vi "Verification.vi"(1 "appended array 2":string[][](array[string])) -> (0 "Array":i32[][](array[numeric]))   [LabVIEW 2019]
panel:
  in  "Blank Button 48":bool
  in  "Blank Button 47":bool
  in  "Blank Button 46":bool
  in  "Blank Button 45":bool
  in  "Blank Button 44":bool
  in  "Blank Button 43":bool
  in  "Blank Button 42":bool
  in  "Blank Button 41":bool
  in  "Color Box 45":u32(colorbox)
  in  "Color Box 46":u32(colorbox)
  in  "Color Box 48":u32(colorbox)
  in  "Color Box 43":u32(colorbox)
  in  "Color Box 41":u32(colorbox)
  in  "Color Box 42":u32(colorbox)
  in  "Color Box 44":u32(colorbox)
  in  "Color Box 47":u32(colorbox)
  in  "Blank Button 40":bool
  in  "Blank Button 39":bool
  in  "Color Box 40":u32(colorbox)
  in  "Color Box 39":u32(colorbox)
  in  "Blank Button 38":bool
  in  "Blank Button 37":bool
  in  "Color Box 38":u32(colorbox)
  in  "Color Box 37":u32(colorbox)
  in  "Blank Button 36":bool
  in  "Blank Button 35":bool
  in  "Color Box 36":u32(colorbox)
  in  "Color Box 35":u32(colorbox)
  in  "Blank Button 34":bool
  in  "Blank Button 33":bool
  in  "Color Box 34":u32(colorbox)
  in  "Color Box 33":u32(colorbox)
  in  "Blank Button 32":bool
  in  "Blank Button 31":bool
  in  "Color Box 32":u32(colorbox)
  in  "Color Box 31":u32(colorbox)
  in  "Blank Button 30":bool
  in  "Blank Button 29":bool
  in  "Color Box 30":u32(colorbox)
  in  "Color Box 29":u32(colorbox)
  in  "Blank Button 28":bool
  in  "Blank Button 27":bool
  in  "Color Box 28":u32(colorbox)
  in  "Color Box 27":u32(colorbox)
  in  "Blank Button 26":bool
  in  "Blank Button 25":bool
  in  "Color Box 26":u32(colorbox)
  in  "Color Box 25":u32(colorbox)
  in  "Blank Button 24":bool
  in  "Blank Button 23":bool
  in  "Blank Button 22":bool
  in  "Blank Button 21":bool
  in  "Blank Button 20":bool
  in  "Blank Button 19":bool
  in  "Blank Button 18":bool
  in  "Blank Button 17":bool
  in  "Color Box 24":u32(colorbox)
  in  "Color Box 22":u32(colorbox)
  in  "Color Box 21":u32(colorbox)
  in  "Color Box 19":u32(colorbox)
  in  "Color Box 23":u32(colorbox)
  in  "Color Box 18":u32(colorbox)
  in  "Color Box 17":u32(colorbox)
  in  "Color Box 20":u32(colorbox)
  in  "Blank Button 16":bool
  in  "Blank Button 15":bool
  in  "Blank Button 14":bool
  in  "Blank Button 13":bool
  in  "Blank Button 12":bool
  in  "Blank Button 11":bool
  in  "Blank Button 10":bool
  in  "Blank Button 9":bool
  in  "Color Box 16":u32(colorbox)
  in  "Color Box 14":u32(colorbox)
  in  "Color Box 11":u32(colorbox)
  in  "Color Box 13":u32(colorbox)
  in  "Color Box 9":u32(colorbox)
  in  "Color Box 15":u32(colorbox)
  in  "Color Box 12":u32(colorbox)
  in  "Color Box 10":u32(colorbox)
  in  "Blank Button 8":bool
  in  "Blank Button 7":bool
  in  "Blank Button 6":bool
  in  "Blank Button 5":bool
  in  "Blank Button 2":bool
  in  "Blank Button":bool
  in  "Color Box 2":u32(colorbox)
  in  "Color Box":u32(colorbox)
  in  "Blank Button 4":bool
  in  "Blank Button 3":bool
  in  "Color Box 4":u32(colorbox)
  in  "Color Box 3":u32(colorbox)
  in  "Color Box 8":u32(colorbox)
  in  "Color Box 5":u32(colorbox)
  in  "Color Box 6":u32(colorbox)
  in  "Color Box 7":u32(colorbox)
  in  "stop":bool
  in  "Blanc":dbl
  in  "Vert":dbl
  in  "Bleu":dbl
  in  "Orange":dbl
  in  "Jaune":dbl
  in  "Rouge":dbl
  # "Vérification des couleurs"
  # "W"
  # "R"
  # "B"
  # "G"
  # "Y"
  # "O"
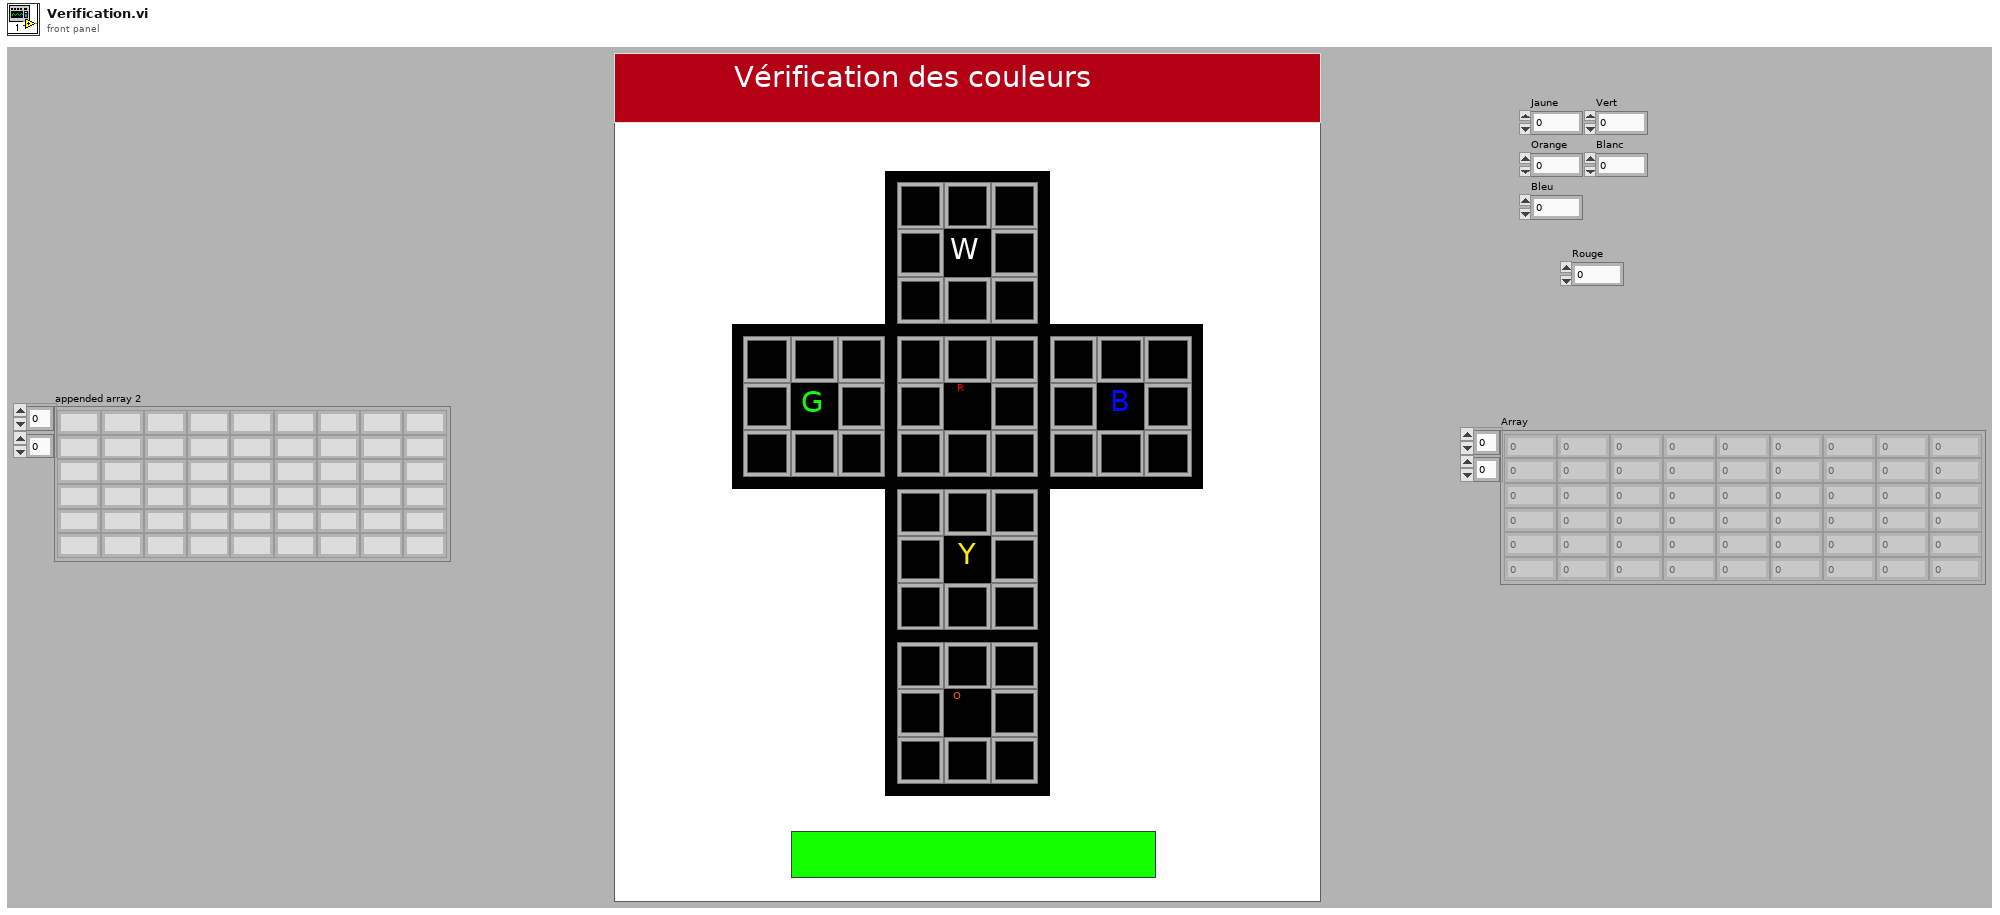
[diagram p1: front panel]
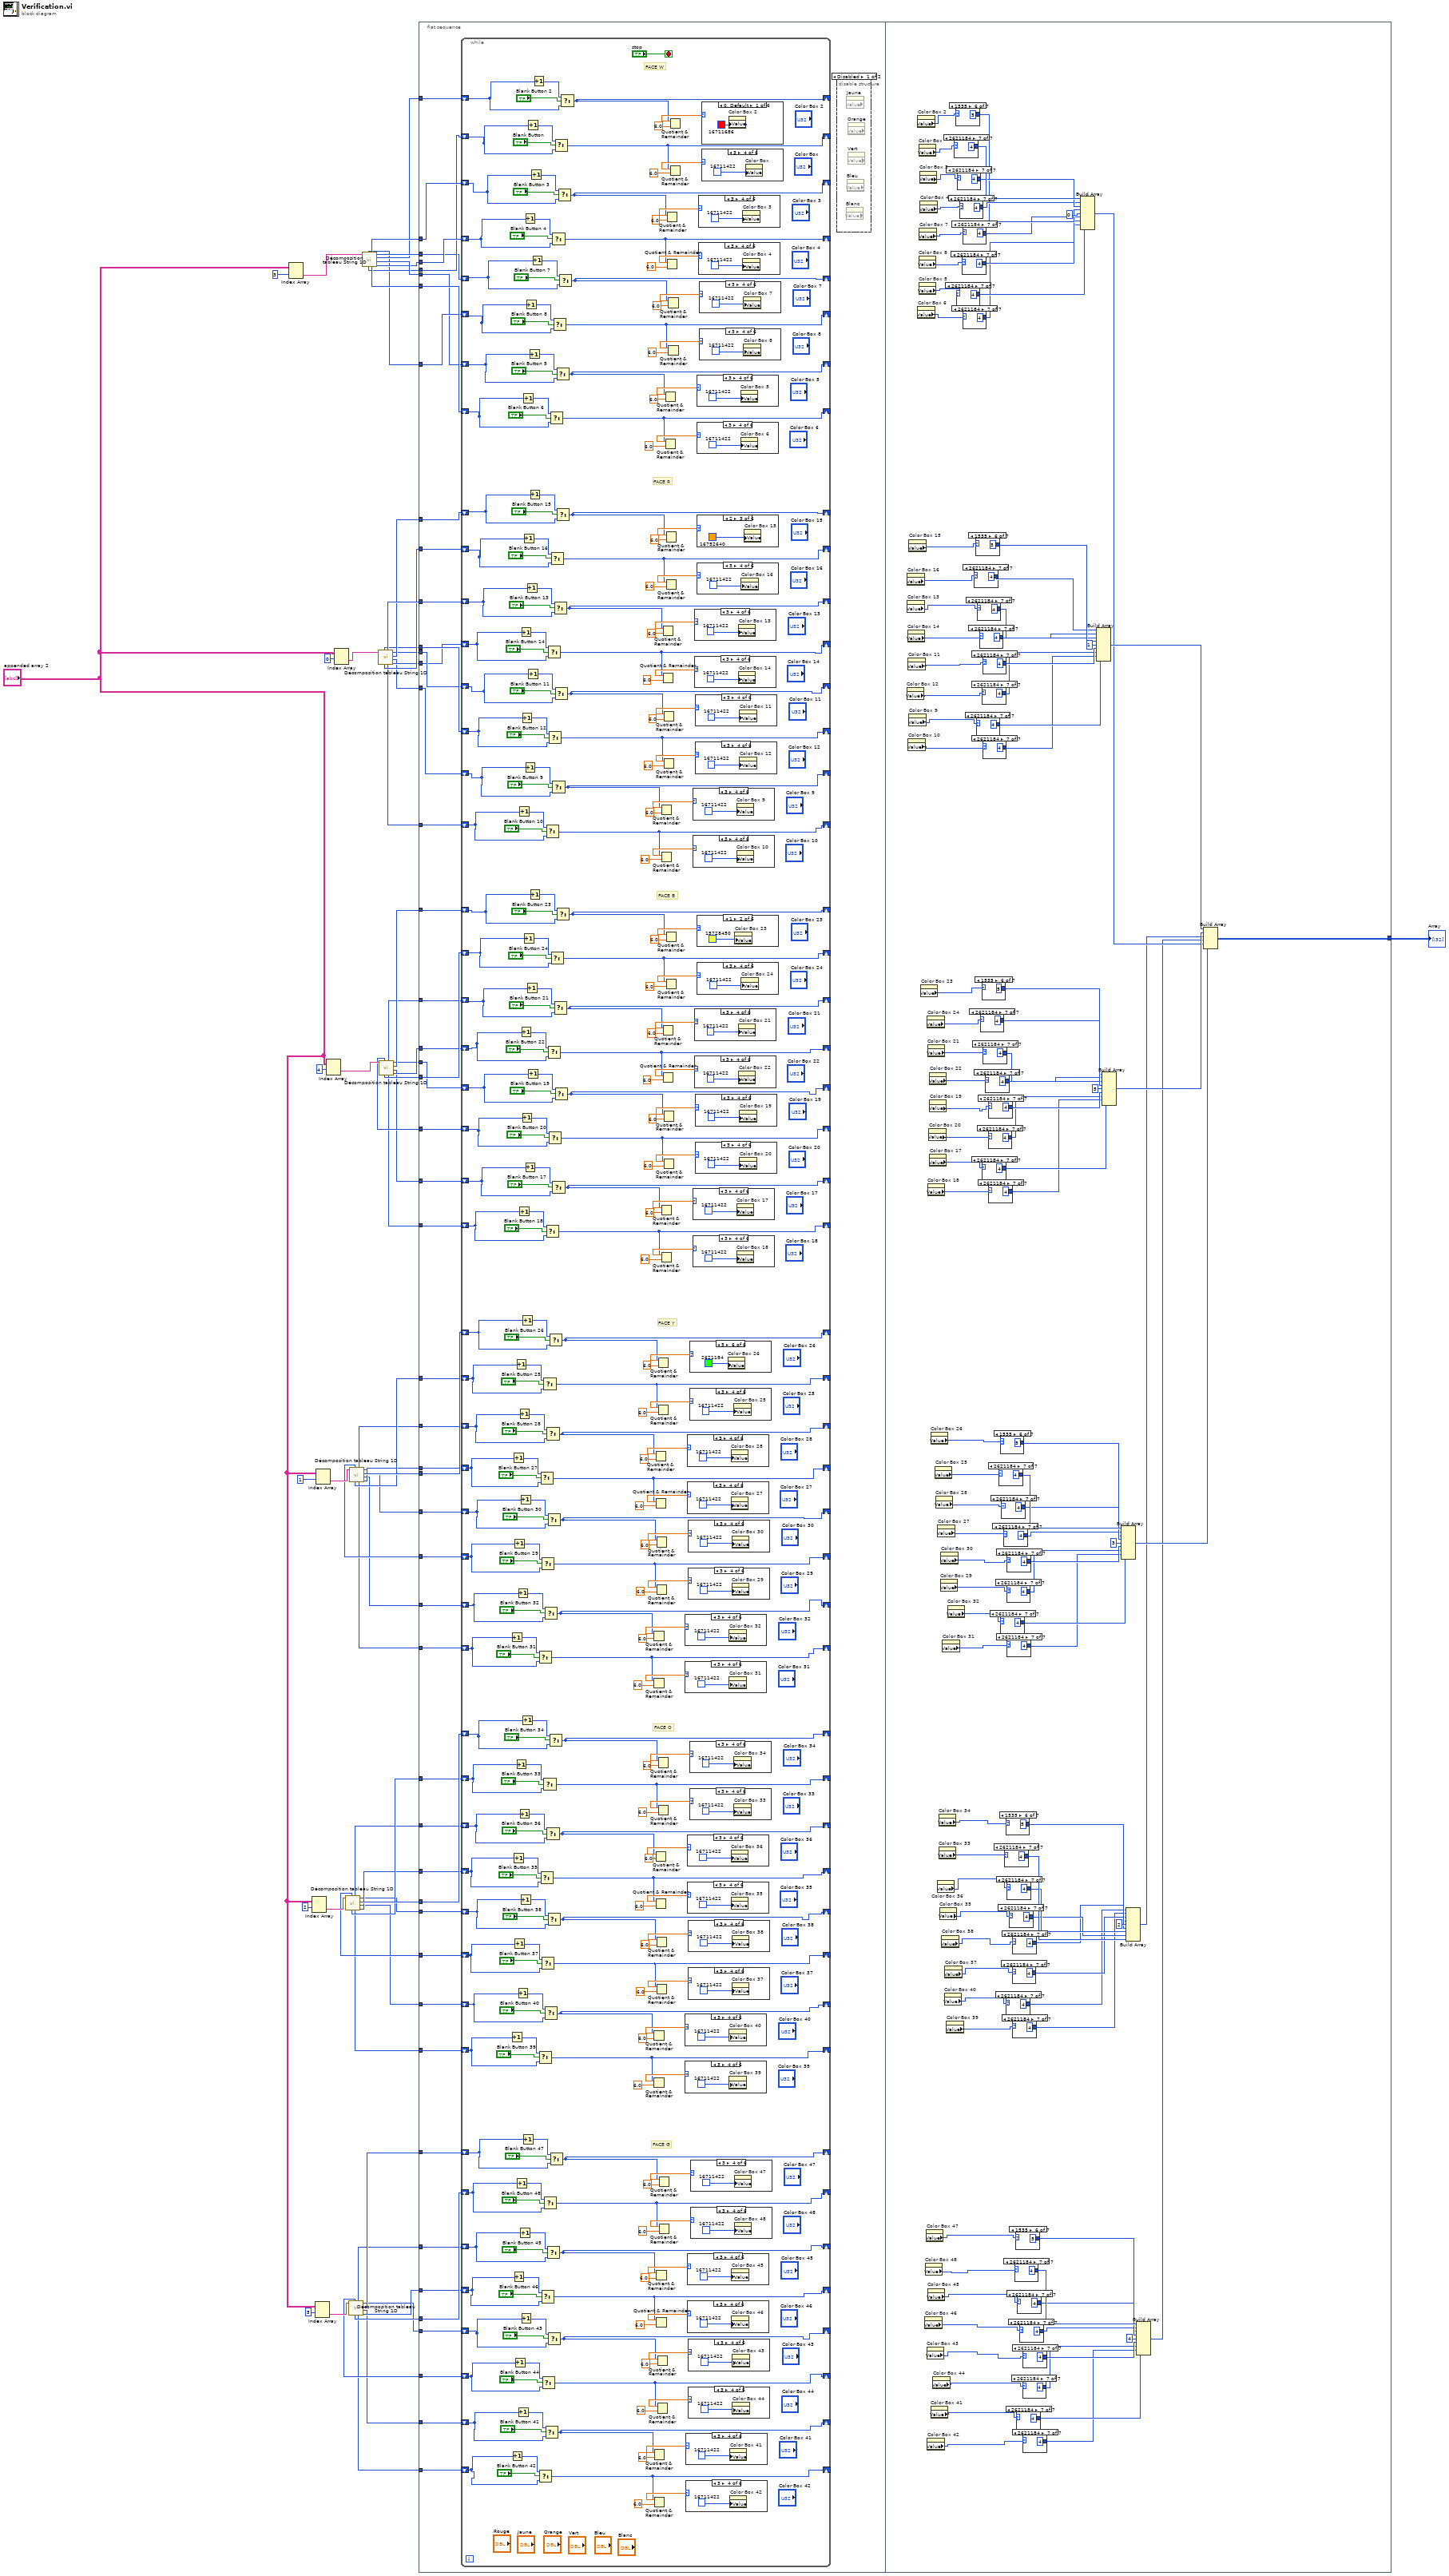
[diagram p0: block diagram]
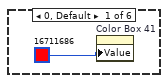
[diagram p3: hidden frame]
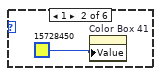
[diagram p4: hidden frame]
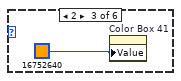
[diagram p5: hidden frame]
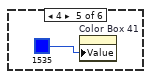
[diagram p6: hidden frame]
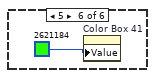
[diagram p7: hidden frame]
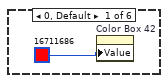
[diagram p8: hidden frame]
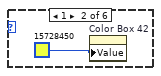
[diagram p9: hidden frame]
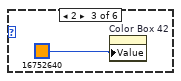
[diagram p10: hidden frame]
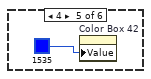
[diagram p11: hidden frame]
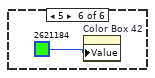
[diagram p12: hidden frame]
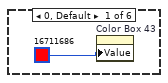
[diagram p13: hidden frame]
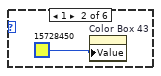
[diagram p14: hidden frame]
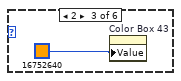
[diagram p15: hidden frame]
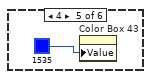
[diagram p16: hidden frame]
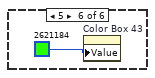
[diagram p17: hidden frame]
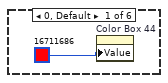
[diagram p18: hidden frame]
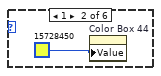
[diagram p19: hidden frame]
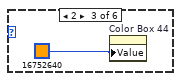
[diagram p20: hidden frame]
diagram:
  n1 = Index Array(array="appended array 2", index (row)=3) -> (element=w61:string[])  [unwired: 1 in]
  n2 = Index Array(array="appended array 2", index (row)=2) -> (element=w37:string[])  [unwired: 1 in]
  n3 = Index Array(array="appended array 2", index (row)=5) -> (element=w38:string[])  [unwired: 1 in]
  n4 = Index Array(array="appended array 2", index (row)=1) -> (element=w36:string[])  [unwired: 1 in]
  n5 = Index Array(array="appended array 2", index (row)=4) -> (element=w41:string[])  [unwired: 1 in]
  n6 = Index Array(array="appended array 2", index (row)=0) -> (element=w52:string[])  [unwired: 1 in]
  n7 = call "Décomposition tableau String 1D.vi"("appended array in"=w37) -> ("7"=w22:i32, "6"=w19:i32, "4"=w25:i32, "3"=w21:i32, "8"=w18:i32, "2"=w23:i32, "9"=w24:i32, "1"=w20:i32)  [unwired: 3 in]
  n8 = call "Décomposition tableau String 1D.vi"("appended array in"=w38) -> ("7"=w30:i32, "6"=w27:i32, "4"=w33:i32, "3"=w29:i32, "8"=w26:i32, "2"=w31:i32, "9"=w32:i32, "1"=w28:i32)  [unwired: 3 in]
  n9 = call "Décomposition tableau String 1D.vi"("appended array in"=w36) -> ("7"=w14:i32, "6"=w11:i32, "4"=w17:i32, "3"=w13:i32, "8"=w10:i32, "2"=w15:i32, "9"=w16:i32, "1"=w12:i32)  [unwired: 3 in]
  n10 = call "Décomposition tableau String 1D.vi"("appended array in"=w61) -> ("7"=w57:i32, "6"=w58:i32, "4"=w54:i32, "3"=w59:i32, "8"=w56:i32, "2"=w60:i32, "9"=w55:i32, "1"=w51:i32)  [unwired: 3 in]
  n11 = call "Décomposition tableau String 1D.vi"("appended array in"=w52) -> ("7"=w47:i32, "6"=w44:i32, "4"=w49:i32, "3"=w46:i32, "8"=w43:i32, "2"=w50:i32, "9"=w48:i32, "1"=w45:i32)  [unwired: 3 in]
  n12 = call "Décomposition tableau String 1D.vi"("appended array in"=w41) -> ("7"=w6:i32, "6"=w3:i32, "4"=w9:i32, "3"=w5:i32, "8"=w2:i32, "2"=w7:i32, "9"=w8:i32, "1"=w4:i32)  [unwired: 3 in]
  n13 = flat-sequence {
    tunnel: w60 -> [w110]
    tunnel: w59 -> [w105]
    tunnel: w57 -> [w109]
    tunnel: w56 -> [w108]
    tunnel: w55 -> [w107]
    tunnel: w54 -> [w106]
    tunnel: w51 -> [w104]
    tunnel: w58 -> [w103]
    tunnel: w43 -> [w102]
    tunnel: w45 -> [w101]
    tunnel: w49 -> [w100]
    tunnel: w48 -> [w99]
    tunnel: w46 -> [w98]
    tunnel: w47 -> [w97]
    tunnel: w50 -> [w96]
    tunnel: w44 -> [w95]
    tunnel: w33 -> [w94]
    tunnel: w32 -> [w93]
    tunnel: w31 -> [w92]
    tunnel: w30 -> [w91]
    tunnel: w29 -> [w90]
    tunnel: w28 -> [w89]
    tunnel: w27 -> [w88]
    tunnel: w26 -> [w87]
    tunnel: w25 -> [w86]
    tunnel: w24 -> [w85]
    tunnel: w23 -> [w84]
    tunnel: w22 -> [w83]
    tunnel: w21 -> [w82]
    tunnel: w20 -> [w81]
    tunnel: w19 -> [w80]
    tunnel: w18 -> [w79]
    tunnel: w17 -> [w78]
    tunnel: w16 -> [w77]
    tunnel: w15 -> [w76]
    tunnel: w14 -> [w75]
    tunnel: w13 -> [w74]
    tunnel: w12 -> [w73]
    tunnel: w11 -> [w72]
    tunnel: w10 -> [w71]
    tunnel: w9 -> [w70]
    tunnel: w8 -> [w69]
    tunnel: w7 -> [w68]
    tunnel: w6 -> [w67]
    tunnel: w5 -> [w66]
    tunnel: w4 -> [w65]
    tunnel: w3 -> [w64]
    tunnel: w2 -> [w63]
    tunnel: [w796] -> w1
    frame #0 {
      n14 = while {
        shift-right: [w392] -> _
        shift-left: w106 -> [w389]
        shift-right: [w390] -> _
        shift-left: w107 -> [w396]
        shift-right: [w377] -> _
        shift-left: w110 -> [w378]
        shift-right: [w375] -> _
        shift-left: w109 -> [w376]
        shift-right: [w356] -> _
        shift-left: w105 -> [w351]
        shift-right: [w355] -> _
        shift-left: w104 -> [w352]
        shift-right: [w354] -> _
        shift-left: w103 -> [w357]
        shift-right: [w353] -> _
        shift-left: w108 -> [w358]
        shift-right: [w317] -> _
        shift-left: w100 -> [w318]
        shift-right: [w316] -> _
        shift-left: w99 -> [w309]
        shift-right: [w315] -> _
        shift-left: w96 -> [w308]
        shift-right: [w314] -> _
        shift-left: w97 -> [w307]
        shift-right: [w313] -> _
        shift-left: w98 -> [w306]
        shift-right: [w312] -> _
        shift-left: w101 -> [w305]
        shift-right: [w311] -> _
        shift-left: w95 -> [w304]
        shift-right: [w310] -> _
        shift-left: w102 -> [w303]
        shift-right: [w270] -> _
        shift-left: w70 -> [w262]
        shift-right: [w269] -> _
        shift-left: w69 -> [w261]
        shift-right: [w268] -> _
        shift-left: w68 -> [w260]
        shift-right: [w267] -> _
        shift-left: w67 -> [w259]
        shift-right: [w266] -> _
        shift-left: w66 -> [w258]
        shift-right: [w265] -> _
        shift-left: w65 -> [w257]
        shift-right: [w264] -> _
        shift-left: w64 -> [w256]
        shift-right: [w263] -> _
        shift-left: w63 -> [w255]
        shift-right: [w168] -> _
        shift-left: w78 -> [w163]
        shift-right: [w167] -> _
        shift-left: w77 -> [w164]
        shift-right: [w166] -> _
        shift-left: w76 -> [w165]
        shift-right: [w169] -> _
        shift-left: w75 -> [w162]
        shift-right: [w170] -> _
        shift-left: w74 -> [w161]
        shift-right: [w171] -> _
        shift-left: w73 -> [w160]
        shift-right: [w172] -> _
        shift-left: w72 -> [w159]
        shift-right: [w173] -> _
        shift-left: w71 -> [w174]
        shift-right: [w189] -> _
        shift-left: w86 -> [w190]
        shift-right: [w188] -> _
        shift-left: w85 -> [w181]
        shift-right: [w187] -> _
        shift-left: w84 -> [w180]
        shift-right: [w186] -> _
        shift-left: w83 -> [w177]
        shift-right: [w185] -> _
        shift-left: w82 -> [w179]
        shift-right: [w184] -> _
        shift-left: w81 -> [w178]
        shift-right: [w183] -> _
        shift-left: w80 -> [w176]
        shift-right: [w182] -> _
        shift-left: w79 -> [w175]
        shift-right: [w126] -> _
        shift-left: w94 -> [w124]
        shift-right: [w123] -> _
        shift-left: w93 -> [w125]
        shift-right: [w122] -> _
        shift-left: w92 -> [w111]
        shift-right: [w121] -> _
        shift-left: w91 -> [w112]
        shift-right: [w120] -> _
        shift-left: w90 -> [w113]
        shift-right: [w119] -> _
        shift-left: w89 -> [w114]
        shift-right: [w118] -> _
        shift-left: w88 -> [w115]
        shift-right: [w117] -> _
        shift-left: w87 -> [w116]
        stop <- "stop" stop-if-true
        # "FACE G"
        # "FACE O"
        # "FACE Y"
        # "FACE B"
        # "FACE R"
        # "FACE W"
        n15 = Increment(x=w174) -> (x+1=w240:i32)
        n16 = Increment(x=w175) -> (x+1=w205:i32)
        n17 = Increment(x=w116) -> (x+1=w144:i32)
        n18 = Increment(x=w162) -> (x+1=w237:i32)
        n19 = Increment(x=w177) -> (x+1=w208:i32)
        n20 = Increment(x=w112) -> (x+1=w141:i32)
        n21 = Increment(x=w160) -> (x+1=w253:i32)
        n22 = Increment(x=w178) -> (x+1=w192:i32)
        n23 = Increment(x=w114) -> (x+1=w157:i32)
        n24 = Increment(x=w164) -> (x+1=w224:i32)
        n25 = Increment(x=w181) -> (x+1=w221:i32)
        n26 = Increment(x=w125) -> (x+1=w128:i32)
        n27 = Increment(x=w159) -> (x+1=w239:i32)
        n28 = Increment(x=w176) -> (x+1=w206:i32)
        n29 = Increment(x=w115) -> (x+1=w143:i32)
        n30 = Increment(x=w303) -> (x+1=w336:i32)
        n31 = Increment(x=w255) -> (x+1=w285:i32)
        n32 = Increment(x=w165) -> (x+1=w238:i32)
        n33 = Increment(x=w180) -> (x+1=w207:i32)
        n34 = Increment(x=w111) -> (x+1=w142:i32)
        n35 = Increment(x=w161) -> (x+1=w254:i32)
        n36 = Increment(x=w179) -> (x+1=w191:i32)
        n37 = Increment(x=w307) -> (x+1=w333:i32)
        n38 = Increment(x=w259) -> (x+1=w288:i32)
        n39 = Increment(x=w113) -> (x+1=w158:i32)
        n40 = Increment(x=w305) -> (x+1=w349:i32)
        n41 = Increment(x=w257) -> (x+1=w272:i32)
        n42 = Increment(x=w163) -> (x+1=w223:i32)
        n43 = Increment(x=w190) -> (x+1=w222:i32)
        n44 = Increment(x=w124) -> (x+1=w127:i32)
        n45 = Increment(x=w358) -> (x+1=w373:i32)
        n46 = Increment(x=w309) -> (x+1=w320:i32)
        n47 = Increment(x=w261) -> (x+1=w301:i32)
        n48 = Increment(x=w376) -> (x+1=w380:i32)
        n49 = Increment(x=w304) -> (x+1=w335:i32)
        n50 = Increment(x=w256) -> (x+1=w286:i32)
        n51 = Increment(x=w352) -> (x+1=w360:i32)
        n52 = Increment(x=w308) -> (x+1=w334:i32)
        n53 = Increment(x=w260) -> (x+1=w287:i32)
        n54 = Increment(x=w396) -> (x+1=w397:i32)
        n55 = Increment(x=w306) -> (x+1=w350:i32)
        n56 = Increment(x=w258) -> (x+1=w271:i32)
        n57 = Increment(x=w357) -> (x+1=w374:i32)
        n58 = Increment(x=w318) -> (x+1=w319:i32)
        n59 = Increment(x=w262) -> (x+1=w302:i32)
        n60 = Increment(x=w378) -> (x+1=w379:i32)
        n61 = Increment(x=w351) -> (x+1=w359:i32)
        n62 = Increment(x=w389) -> (x+1=w398:i32)
        n63 = Select(t=w240, s="Blank Button 31", f=w174) -> (s? t:f=w173:i32)
        n64 = Select(t=w205, s="Blank Button 39", f=w175) -> (s? t:f=w182:i32)
        n65 = Select(t=w144, s="Blank Button 42", f=w116) -> (s? t:f=w117:i32)
        n66 = Select(t=w237, s="Blank Button 27", f=w162) -> (s? t:f=w169:i32)
        n67 = Select(t=w208, s="Blank Button 35", f=w177) -> (s? t:f=w186:i32)
        n68 = Select(t=w141, s="Blank Button 46", f=w112) -> (s? t:f=w121:i32)
        n69 = Select(t=w253, s="Blank Button 29", f=w160) -> (s? t:f=w171:i32)
        n70 = Select(t=w192, s="Blank Button 37", f=w178) -> (s? t:f=w184:i32)
        n71 = Select(t=w157, s="Blank Button 44", f=w114) -> (s? t:f=w119:i32)
        n72 = Select(t=w224, s="Blank Button 25", f=w164) -> (s? t:f=w167:i32)
        n73 = Select(t=w221, s="Blank Button 33", f=w181) -> (s? t:f=w188:i32)
        n74 = Select(t=w128, s="Blank Button 48", f=w125) -> (s? t:f=w123:i32)
        n75 = Select(t=w239, s="Blank Button 32", f=w159) -> (s? t:f=w172:i32)
        n76 = Select(t=w206, s="Blank Button 40", f=w176) -> (s? t:f=w183:i32)
        n77 = Select(t=w143, s="Blank Button 41", f=w115) -> (s? t:f=w118:i32)
        n78 = Select(t=w336, s="Blank Button 10", f=w303) -> (s? t:f=w310:i32)
        n79 = Select(t=w285, s="Blank Button 18", f=w255) -> (s? t:f=w263:i32)
        n80 = Select(t=w238, s="Blank Button 28", f=w165) -> (s? t:f=w166:i32)
        n81 = Select(t=w207, s="Blank Button 36", f=w180) -> (s? t:f=w187:i32)
        n82 = Select(t=w142, s="Blank Button 45", f=w111) -> (s? t:f=w122:i32)
        n83 = Select(t=w254, s="Blank Button 30", f=w161) -> (s? t:f=w170:i32)
        n84 = Select(t=w191, s="Blank Button 38", f=w179) -> (s? t:f=w185:i32)
        n85 = Select(t=w333, s="Blank Button 14", f=w307) -> (s? t:f=w314:i32)
        n86 = Select(t=w288, s="Blank Button 22", f=w259) -> (s? t:f=w267:i32)
        n87 = Select(t=w158, s="Blank Button 43", f=w113) -> (s? t:f=w120:i32)
        n88 = Select(t=w349, s="Blank Button 12", f=w305) -> (s? t:f=w312:i32)
        n89 = Select(t=w272, s="Blank Button 20", f=w257) -> (s? t:f=w265:i32)
        n90 = Select(t=w223, s="Blank Button 26", f=w163) -> (s? t:f=w168:i32)
        n91 = Select(t=w222, s="Blank Button 34", f=w190) -> (s? t:f=w189:i32)
        n92 = Select(t=w127, s="Blank Button 47", f=w124) -> (s? t:f=w126:i32)
        n93 = Select(t=w373, s="Blank Button 6", f=w358) -> (s? t:f=w353:i32)
        n94 = Select(t=w320, s="Blank Button 16", f=w309) -> (s? t:f=w316:i32)
        n95 = Select(t=w301, s="Blank Button 24", f=w261) -> (s? t:f=w269:i32)
        n96 = Select(t=w380, s="Blank Button 4", f=w376) -> (s? t:f=w375:i32)
        n97 = Select(t=w335, s="Blank Button 9", f=w304) -> (s? t:f=w311:i32)
        n98 = Select(t=w286, s="Blank Button 17", f=w256) -> (s? t:f=w264:i32)
        n99 = Select(t=w360, s="Blank Button 8", f=w352) -> (s? t:f=w355:i32)
        n100 = Select(t=w334, s="Blank Button 13", f=w308) -> (s? t:f=w315:i32)
        n101 = Select(t=w287, s="Blank Button 21", f=w260) -> (s? t:f=w268:i32)
        n102 = Select(t=w397, s="Blank Button", f=w396) -> (s? t:f=w390:i32)
        n103 = Select(t=w350, s="Blank Button 11", f=w306) -> (s? t:f=w313:i32)
        n104 = Select(t=w271, s="Blank Button 19", f=w258) -> (s? t:f=w266:i32)
        n105 = Select(t=w374, s="Blank Button 5", f=w357) -> (s? t:f=w354:i32)
        n106 = Select(t=w319, s="Blank Button 15", f=w318) -> (s? t:f=w317:i32)
        n107 = Select(t=w302, s="Blank Button 23", f=w262) -> (s? t:f=w270:i32)
        n108 = Select(t=w379, s="Blank Button 3", f=w378) -> (s? t:f=w377:i32)
        n109 = Select(t=w359, s="Blank Button 7", f=w351) -> (s? t:f=w356:i32)
        n110 = Select(t=w398, s="Blank Button 2", f=w389) -> (s? t:f=w392:i32)
        n111 = Quotient & Remainder(x=w172, y=6.0) -> (x-y*floor(x/y)=w243:dbl)  [unwired: 1 out]
        n112 = Quotient & Remainder(x=w173, y=6.0) -> (x-y*floor(x/y)=w241:dbl)  [unwired: 1 out]
        n113 = Quotient & Remainder(x=w183, y=6.0) -> (x-y*floor(x/y)=w202:dbl)  [unwired: 1 out]
        n114 = Quotient & Remainder(x=w182, y=6.0) -> (x-y*floor(x/y)=w204:dbl)  [unwired: 1 out]
        n115 = Quotient & Remainder(x=w118, y=6.0) -> (x-y*floor(x/y)=w147:dbl)  [unwired: 1 out]
        n116 = Quotient & Remainder(x=w117, y=6.0) -> (x-y*floor(x/y)=w145:dbl)  [unwired: 1 out]
        n117 = Quotient & Remainder(x=w166, y=6.0) -> (x-y*floor(x/y)=w234:dbl)  [unwired: 1 out]
        n118 = Quotient & Remainder(x=w169, y=6.0) -> (x-y*floor(x/y)=w236:dbl)  [unwired: 1 out]
        n119 = Quotient & Remainder(x=w187, y=6.0) -> (x-y*floor(x/y)=w211:dbl)  [unwired: 1 out]
        n120 = Quotient & Remainder(x=w186, y=6.0) -> (x-y*floor(x/y)=w209:dbl)  [unwired: 1 out]
        n121 = Quotient & Remainder(x=w122, y=6.0) -> (x-y*floor(x/y)=w138:dbl)  [unwired: 1 out]
        n122 = Quotient & Remainder(x=w121, y=6.0) -> (x-y*floor(x/y)=w140:dbl)  [unwired: 1 out]
        n123 = Quotient & Remainder(x=w170, y=6.0) -> (x-y*floor(x/y)=w250:dbl)  [unwired: 1 out]
        n124 = Quotient & Remainder(x=w171, y=6.0) -> (x-y*floor(x/y)=w252:dbl)  [unwired: 1 out]
        n125 = Quotient & Remainder(x=w185, y=6.0) -> (x-y*floor(x/y)=w195:dbl)  [unwired: 1 out]
        n126 = Quotient & Remainder(x=w184, y=6.0) -> (x-y*floor(x/y)=w193:dbl)  [unwired: 1 out]
        n127 = Quotient & Remainder(x=w120, y=6.0) -> (x-y*floor(x/y)=w154:dbl)  [unwired: 1 out]
        n128 = Quotient & Remainder(x=w119, y=6.0) -> (x-y*floor(x/y)=w156:dbl)  [unwired: 1 out]
        n129 = Quotient & Remainder(x=w168, y=6.0) -> (x-y*floor(x/y)=w227:dbl)  [unwired: 1 out]
        n130 = Quotient & Remainder(x=w167, y=6.0) -> (x-y*floor(x/y)=w225:dbl)  [unwired: 1 out]
        n131 = Quotient & Remainder(x=w189, y=6.0) -> (x-y*floor(x/y)=w218:dbl)  [unwired: 1 out]
        n132 = Quotient & Remainder(x=w188, y=6.0) -> (x-y*floor(x/y)=w220:dbl)  [unwired: 1 out]
        n133 = Quotient & Remainder(x=w126, y=6.0) -> (x-y*floor(x/y)=w131:dbl)  [unwired: 1 out]
        n134 = Quotient & Remainder(x=w123, y=6.0) -> (x-y*floor(x/y)=w129:dbl)  [unwired: 1 out]
        n135 = Quotient & Remainder(x=w311, y=6.0) -> (x-y*floor(x/y)=w339:dbl)  [unwired: 1 out]
        n136 = Quotient & Remainder(x=w310, y=6.0) -> (x-y*floor(x/y)=w337:dbl)  [unwired: 1 out]
        n137 = Quotient & Remainder(x=w264, y=6.0) -> (x-y*floor(x/y)=w282:dbl)  [unwired: 1 out]
        n138 = Quotient & Remainder(x=w263, y=6.0) -> (x-y*floor(x/y)=w284:dbl)  [unwired: 1 out]
        n139 = Quotient & Remainder(x=w315, y=6.0) -> (x-y*floor(x/y)=w330:dbl)  [unwired: 1 out]
        n140 = Quotient & Remainder(x=w314, y=6.0) -> (x-y*floor(x/y)=w332:dbl)  [unwired: 1 out]
        n141 = Quotient & Remainder(x=w268, y=6.0) -> (x-y*floor(x/y)=w291:dbl)  [unwired: 1 out]
        n142 = Quotient & Remainder(x=w267, y=6.0) -> (x-y*floor(x/y)=w289:dbl)  [unwired: 1 out]
        n143 = Quotient & Remainder(x=w313, y=6.0) -> (x-y*floor(x/y)=w346:dbl)  [unwired: 1 out]
        n144 = Quotient & Remainder(x=w312, y=6.0) -> (x-y*floor(x/y)=w348:dbl)  [unwired: 1 out]
        n145 = Quotient & Remainder(x=w266, y=6.0) -> (x-y*floor(x/y)=w275:dbl)  [unwired: 1 out]
        n146 = Quotient & Remainder(x=w265, y=6.0) -> (x-y*floor(x/y)=w273:dbl)  [unwired: 1 out]
        n147 = Quotient & Remainder(x=w354, y=6.0) -> (x-y*floor(x/y)=w370:dbl)  [unwired: 1 out]
        n148 = Quotient & Remainder(x=w353, y=6.0) -> (x-y*floor(x/y)=w372:dbl)  [unwired: 1 out]
        n149 = Quotient & Remainder(x=w317, y=6.0) -> (x-y*floor(x/y)=w323:dbl)  [unwired: 1 out]
        n150 = Quotient & Remainder(x=w316, y=6.0) -> (x-y*floor(x/y)=w321:dbl)  [unwired: 1 out]
        n151 = Quotient & Remainder(x=w270, y=6.0) -> (x-y*floor(x/y)=w298:dbl)  [unwired: 1 out]
        n152 = Quotient & Remainder(x=w269, y=6.0) -> (x-y*floor(x/y)=w300:dbl)  [unwired: 1 out]
        n153 = Quotient & Remainder(x=w377, y=6.0) -> (x-y*floor(x/y)=w383:dbl)  [unwired: 1 out]
        n154 = Quotient & Remainder(x=w375, y=6.0) -> (x-y*floor(x/y)=w381:dbl)  [unwired: 1 out]
        n155 = Quotient & Remainder(x=w356, y=6.0) -> (x-y*floor(x/y)=w363:dbl)  [unwired: 1 out]
        n156 = Quotient & Remainder(x=w355, y=6.0) -> (x-y*floor(x/y)=w361:dbl)  [unwired: 1 out]
        n157 = Quotient & Remainder(x=w392, y=6.0) -> (x-y*floor(x/y)=w393:dbl)  [unwired: 1 out]
        n158 = Quotient & Remainder(x=w390, y=6.0) -> (x-y*floor(x/y)=w395:dbl)  [unwired: 1 out]
        n159 = case shown="3" w243 {
          frame 0, Default {
            n160 = property on="Color Box 32" class="ColBox"("Value"=u32 16711686 ("Color Box")) -> ()  [unwired: 2 in, 2 out]
          }
          frame 1 {
            n161 = property on="Color Box 32" class="ColBox"("Value"=u32 15728450 ("Color Box")) -> ()  [unwired: 2 in, 2 out]
          }
          frame 2 {
            n162 = property on="Color Box 32" class="ColBox"("Value"=u32 16752640 ("Color Box")) -> ()  [unwired: 2 in, 2 out]
          }
          frame 3 {
            n163 = property on="Color Box 32" class="ColBox"("Value"=u32 16711422 ("Color Box")) -> ()  [unwired: 2 in, 2 out]
          }
          frame 4 {
            n164 = property on="Color Box 32" class="ColBox"("Value"=u32 1535 ("Color Box")) -> ()  [unwired: 2 in, 2 out]
          }
          frame 5 {
            n165 = property on="Color Box 32" class="ColBox"("Value"=u32 2621184 ("Color Box")) -> ()  [unwired: 2 in, 2 out]
          }
        }
        n166 = case shown="3" w241 {
          frame 0, Default {
            n167 = property on="Color Box 31" class="ColBox"("Value"=u32 16711686 ("Color Box")) -> ()  [unwired: 2 in, 2 out]
          }
          frame 1 {
            n168 = property on="Color Box 31" class="ColBox"("Value"=u32 15728450 ("Color Box")) -> ()  [unwired: 2 in, 2 out]
          }
          frame 2 {
            n169 = property on="Color Box 31" class="ColBox"("Value"=u32 16752640 ("Color Box")) -> ()  [unwired: 2 in, 2 out]
          }
          frame 3 {
            n170 = property on="Color Box 31" class="ColBox"("Value"=u32 16711422 ("Color Box")) -> ()  [unwired: 2 in, 2 out]
          }
          frame 4 {
            n171 = property on="Color Box 31" class="ColBox"("Value"=u32 1535 ("Color Box")) -> ()  [unwired: 2 in, 2 out]
          }
          frame 5 {
            n172 = property on="Color Box 31" class="ColBox"("Value"=u32 2621184 ("Color Box")) -> ()  [unwired: 2 in, 2 out]
          }
        }
        n173 = case shown="3" w202 {
          frame 0, Default {
            n174 = property on="Color Box 40" class="ColBox"("Value"=u32 16711686 ("Color Box")) -> ()  [unwired: 2 in, 2 out]
          }
          frame 1 {
            n175 = property on="Color Box 40" class="ColBox"("Value"=u32 15728450 ("Color Box")) -> ()  [unwired: 2 in, 2 out]
          }
          frame 2 {
            n176 = property on="Color Box 40" class="ColBox"("Value"=u32 16752640 ("Color Box")) -> ()  [unwired: 2 in, 2 out]
          }
          frame 3 {
            n177 = property on="Color Box 40" class="ColBox"("Value"=u32 16711422 ("Color Box")) -> ()  [unwired: 2 in, 2 out]
          }
          frame 4 {
            n178 = property on="Color Box 40" class="ColBox"("Value"=u32 1535 ("Color Box")) -> ()  [unwired: 2 in, 2 out]
          }
          frame 5 {
            n179 = property on="Color Box 40" class="ColBox"("Value"=u32 2621184 ("Color Box")) -> ()  [unwired: 2 in, 2 out]
          }
        }
        n180 = case shown="3" w204 {
          frame 0, Default {
            n181 = property on="Color Box 39" class="ColBox"("Value"=u32 16711686 ("Color Box")) -> ()  [unwired: 2 in, 2 out]
          }
          frame 1 {
            n182 = property on="Color Box 39" class="ColBox"("Value"=u32 15728450 ("Color Box")) -> ()  [unwired: 2 in, 2 out]
          }
          frame 2 {
            n183 = property on="Color Box 39" class="ColBox"("Value"=u32 16752640 ("Color Box")) -> ()  [unwired: 2 in, 2 out]
          }
          frame 3 {
            n184 = property on="Color Box 39" class="ColBox"("Value"=u32 16711422 ("Color Box")) -> ()  [unwired: 2 in, 2 out]
          }
          frame 4 {
            n185 = property on="Color Box 39" class="ColBox"("Value"=u32 1535 ("Color Box")) -> ()  [unwired: 2 in, 2 out]
          }
          frame 5 {
            n186 = property on="Color Box 39" class="ColBox"("Value"=u32 2621184 ("Color Box")) -> ()  [unwired: 2 in, 2 out]
          }
        }
        n187 = case shown="3" w147 {
          frame 0, Default {
            n188 = property on="Color Box 41" class="ColBox"("Value"=u32 16711686 ("Color Box")) -> ()  [unwired: 2 in, 2 out]
          }
          frame 1 {
            n189 = property on="Color Box 41" class="ColBox"("Value"=u32 15728450 ("Color Box")) -> ()  [unwired: 2 in, 2 out]
          }
          frame 2 {
            n190 = property on="Color Box 41" class="ColBox"("Value"=u32 16752640 ("Color Box")) -> ()  [unwired: 2 in, 2 out]
          }
          frame 3 {
            n191 = property on="Color Box 41" class="ColBox"("Value"=u32 16711422 ("Color Box")) -> ()  [unwired: 2 in, 2 out]
          }
          frame 4 {
            n192 = property on="Color Box 41" class="ColBox"("Value"=u32 1535 ("Color Box")) -> ()  [unwired: 2 in, 2 out]
          }
          frame 5 {
            n193 = property on="Color Box 41" class="ColBox"("Value"=u32 2621184 ("Color Box")) -> ()  [unwired: 2 in, 2 out]
          }
        }
        n194 = case shown="3" w145 {
          frame 0, Default {
            n195 = property on="Color Box 42" class="ColBox"("Value"=u32 16711686 ("Color Box")) -> ()  [unwired: 2 in, 2 out]
          }
          frame 1 {
            n196 = property on="Color Box 42" class="ColBox"("Value"=u32 15728450 ("Color Box")) -> ()  [unwired: 2 in, 2 out]
          }
          frame 2 {
            n197 = property on="Color Box 42" class="ColBox"("Value"=u32 16752640 ("Color Box")) -> ()  [unwired: 2 in, 2 out]
          }
          frame 3 {
            n198 = property on="Color Box 42" class="ColBox"("Value"=u32 16711422 ("Color Box")) -> ()  [unwired: 2 in, 2 out]
          }
          frame 4 {
            n199 = property on="Color Box 42" class="ColBox"("Value"=u32 1535 ("Color Box")) -> ()  [unwired: 2 in, 2 out]
          }
          frame 5 {
            n200 = property on="Color Box 42" class="ColBox"("Value"=u32 2621184 ("Color Box")) -> ()  [unwired: 2 in, 2 out]
          }
        }
        n201 = case shown="3" w234 {
          frame 0, Default {
            n202 = property on="Color Box 28" class="ColBox"("Value"=u32 16711686 ("Color Box")) -> ()  [unwired: 2 in, 2 out]
          }
          frame 1 {
            n203 = property on="Color Box 28" class="ColBox"("Value"=u32 15728450 ("Color Box")) -> ()  [unwired: 2 in, 2 out]
          }
          frame 2 {
            n204 = property on="Color Box 28" class="ColBox"("Value"=u32 16752640 ("Color Box")) -> ()  [unwired: 2 in, 2 out]
          }
          frame 3 {
            n205 = property on="Color Box 28" class="ColBox"("Value"=u32 16711422 ("Color Box")) -> ()  [unwired: 2 in, 2 out]
          }
          frame 4 {
            n206 = property on="Color Box 28" class="ColBox"("Value"=u32 1535 ("Color Box")) -> ()  [unwired: 2 in, 2 out]
          }
          frame 5 {
            n207 = property on="Color Box 28" class="ColBox"("Value"=u32 2621184 ("Color Box")) -> ()  [unwired: 2 in, 2 out]
          }
        }
        n208 = case shown="3" w236 {
          frame 0, Default {
            n209 = property on="Color Box 27" class="ColBox"("Value"=u32 16711686 ("Color Box")) -> ()  [unwired: 2 in, 2 out]
          }
          frame 1 {
            n210 = property on="Color Box 27" class="ColBox"("Value"=u32 15728450 ("Color Box")) -> ()  [unwired: 2 in, 2 out]
          }
          frame 2 {
            n211 = property on="Color Box 27" class="ColBox"("Value"=u32 16752640 ("Color Box")) -> ()  [unwired: 2 in, 2 out]
          }
          frame 3 {
            n212 = property on="Color Box 27" class="ColBox"("Value"=u32 16711422 ("Color Box")) -> ()  [unwired: 2 in, 2 out]
          }
          frame 4 {
            n213 = property on="Color Box 27" class="ColBox"("Value"=u32 1535 ("Color Box")) -> ()  [unwired: 2 in, 2 out]
          }
          frame 5 {
            n214 = property on="Color Box 27" class="ColBox"("Value"=u32 2621184 ("Color Box")) -> ()  [unwired: 2 in, 2 out]
          }
        }
        n215 = case shown="3" w211 {
          frame 0, Default {
            n216 = property on="Color Box 36" class="ColBox"("Value"=u32 16711686 ("Color Box")) -> ()  [unwired: 2 in, 2 out]
          }
          frame 1 {
            n217 = property on="Color Box 36" class="ColBox"("Value"=u32 15728450 ("Color Box")) -> ()  [unwired: 2 in, 2 out]
          }
          frame 2 {
            n218 = property on="Color Box 36" class="ColBox"("Value"=u32 16752640 ("Color Box")) -> ()  [unwired: 2 in, 2 out]
          }
          frame 3 {
            n219 = property on="Color Box 36" class="ColBox"("Value"=u32 16711422 ("Color Box")) -> ()  [unwired: 2 in, 2 out]
          }
          frame 4 {
            n220 = property on="Color Box 36" class="ColBox"("Value"=u32 1535 ("Color Box")) -> ()  [unwired: 2 in, 2 out]
          }
          frame 5 {
            n221 = property on="Color Box 36" class="ColBox"("Value"=u32 2621184 ("Color Box")) -> ()  [unwired: 2 in, 2 out]
          }
        }
        n222 = case shown="3" w209 {
          frame 0, Default {
            n223 = property on="Color Box 35" class="ColBox"("Value"=u32 16711686 ("Color Box")) -> ()  [unwired: 2 in, 2 out]
          }
          frame 1 {
            n224 = property on="Color Box 35" class="ColBox"("Value"=u32 15728450 ("Color Box")) -> ()  [unwired: 2 in, 2 out]
          }
          frame 2 {
            n225 = property on="Color Box 35" class="ColBox"("Value"=u32 16752640 ("Color Box")) -> ()  [unwired: 2 in, 2 out]
          }
          frame 3 {
            n226 = property on="Color Box 35" class="ColBox"("Value"=u32 16711422 ("Color Box")) -> ()  [unwired: 2 in, 2 out]
          }
          frame 4 {
            n227 = property on="Color Box 35" class="ColBox"("Value"=u32 1535 ("Color Box")) -> ()  [unwired: 2 in, 2 out]
          }
          frame 5 {
            n228 = property on="Color Box 35" class="ColBox"("Value"=u32 2621184 ("Color Box")) -> ()  [unwired: 2 in, 2 out]
          }
        }
        n229 = case shown="3" w138 {
          frame 0, Default {
            n230 = property on="Color Box 45" class="ColBox"("Value"=u32 16711686 ("Color Box")) -> ()  [unwired: 2 in, 2 out]
          }
          frame 1 {
            n231 = property on="Color Box 45" class="ColBox"("Value"=u32 15728450 ("Color Box")) -> ()  [unwired: 2 in, 2 out]
          }
          frame 2 {
            n232 = property on="Color Box 45" class="ColBox"("Value"=u32 16752640 ("Color Box")) -> ()  [unwired: 2 in, 2 out]
          }
          frame 3 {
            n233 = property on="Color Box 45" class="ColBox"("Value"=u32 16711422 ("Color Box")) -> ()  [unwired: 2 in, 2 out]
          }
          frame 4 {
            n234 = property on="Color Box 45" class="ColBox"("Value"=u32 1535 ("Color Box")) -> ()  [unwired: 2 in, 2 out]
          }
          frame 5 {
            n235 = property on="Color Box 45" class="ColBox"("Value"=u32 2621184 ("Color Box")) -> ()  [unwired: 2 in, 2 out]
          }
        }
        n236 = case shown="3" w140 {
          frame 0, Default {
            n237 = property on="Color Box 46" class="ColBox"("Value"=u32 16711686 ("Color Box")) -> ()  [unwired: 2 in, 2 out]
          }
          frame 1 {
            n238 = property on="Color Box 46" class="ColBox"("Value"=u32 15728450 ("Color Box")) -> ()  [unwired: 2 in, 2 out]
          }
          frame 2 {
            n239 = property on="Color Box 46" class="ColBox"("Value"=u32 16752640 ("Color Box")) -> ()  [unwired: 2 in, 2 out]
          }
          frame 3 {
            n240 = property on="Color Box 46" class="ColBox"("Value"=u32 16711422 ("Color Box")) -> ()  [unwired: 2 in, 2 out]
          }
          frame 4 {
            n241 = property on="Color Box 46" class="ColBox"("Value"=u32 1535 ("Color Box")) -> ()  [unwired: 2 in, 2 out]
          }
          frame 5 {
            n242 = property on="Color Box 46" class="ColBox"("Value"=u32 2621184 ("Color Box")) -> ()  [unwired: 2 in, 2 out]
          }
        }
        n243 = case shown="3" w250 {
          frame 0, Default {
            n244 = property on="Color Box 30" class="ColBox"("Value"=u32 16711686 ("Color Box")) -> ()  [unwired: 2 in, 2 out]
          }
          frame 1 {
            n245 = property on="Color Box 30" class="ColBox"("Value"=u32 15728450 ("Color Box")) -> ()  [unwired: 2 in, 2 out]
          }
          frame 2 {
            n246 = property on="Color Box 30" class="ColBox"("Value"=u32 16752640 ("Color Box")) -> ()  [unwired: 2 in, 2 out]
          }
          frame 3 {
            n247 = property on="Color Box 30" class="ColBox"("Value"=u32 16711422 ("Color Box")) -> ()  [unwired: 2 in, 2 out]
          }
          frame 4 {
            n248 = property on="Color Box 30" class="ColBox"("Value"=u32 1535 ("Color Box")) -> ()  [unwired: 2 in, 2 out]
          }
          frame 5 {
            n249 = property on="Color Box 30" class="ColBox"("Value"=u32 2621184 ("Color Box")) -> ()  [unwired: 2 in, 2 out]
          }
        }
        n250 = case shown="3" w252 {
          frame 0, Default {
            n251 = property on="Color Box 29" class="ColBox"("Value"=u32 16711686 ("Color Box")) -> ()  [unwired: 2 in, 2 out]
          }
          frame 1 {
            n252 = property on="Color Box 29" class="ColBox"("Value"=u32 15728450 ("Color Box")) -> ()  [unwired: 2 in, 2 out]
          }
          frame 2 {
            n253 = property on="Color Box 29" class="ColBox"("Value"=u32 16752640 ("Color Box")) -> ()  [unwired: 2 in, 2 out]
          }
          frame 3 {
            n254 = property on="Color Box 29" class="ColBox"("Value"=u32 16711422 ("Color Box")) -> ()  [unwired: 2 in, 2 out]
          }
          frame 4 {
            n255 = property on="Color Box 29" class="ColBox"("Value"=u32 1535 ("Color Box")) -> ()  [unwired: 2 in, 2 out]
          }
          frame 5 {
            n256 = property on="Color Box 29" class="ColBox"("Value"=u32 2621184 ("Color Box")) -> ()  [unwired: 2 in, 2 out]
          }
        }
        n257 = case shown="3" w195 {
          frame 0, Default {
            n258 = property on="Color Box 38" class="ColBox"("Value"=u32 16711686 ("Color Box")) -> ()  [unwired: 2 in, 2 out]
          }
          frame 1 {
            n259 = property on="Color Box 38" class="ColBox"("Value"=u32 15728450 ("Color Box")) -> ()  [unwired: 2 in, 2 out]
          }
          frame 2 {
            n260 = property on="Color Box 38" class="ColBox"("Value"=u32 16752640 ("Color Box")) -> ()  [unwired: 2 in, 2 out]
          }
          frame 3 {
            n261 = property on="Color Box 38" class="ColBox"("Value"=u32 16711422 ("Color Box")) -> ()  [unwired: 2 in, 2 out]
          }
          frame 4 {
            n262 = property on="Color Box 38" class="ColBox"("Value"=u32 1535 ("Color Box")) -> ()  [unwired: 2 in, 2 out]
          }
          frame 5 {
            n263 = property on="Color Box 38" class="ColBox"("Value"=u32 2621184 ("Color Box")) -> ()  [unwired: 2 in, 2 out]
          }
        }
        n264 = case shown="3" w193 {
          frame 0, Default {
            n265 = property on="Color Box 37" class="ColBox"("Value"=u32 16711686 ("Color Box")) -> ()  [unwired: 2 in, 2 out]
          }
          frame 1 {
            n266 = property on="Color Box 37" class="ColBox"("Value"=u32 15728450 ("Color Box")) -> ()  [unwired: 2 in, 2 out]
          }
          frame 2 {
            n267 = property on="Color Box 37" class="ColBox"("Value"=u32 16752640 ("Color Box")) -> ()  [unwired: 2 in, 2 out]
          }
          frame 3 {
            n268 = property on="Color Box 37" class="ColBox"("Value"=u32 16711422 ("Color Box")) -> ()  [unwired: 2 in, 2 out]
          }
          frame 4 {
            n269 = property on="Color Box 37" class="ColBox"("Value"=u32 1535 ("Color Box")) -> ()  [unwired: 2 in, 2 out]
          }
          frame 5 {
            n270 = property on="Color Box 37" class="ColBox"("Value"=u32 2621184 ("Color Box")) -> ()  [unwired: 2 in, 2 out]
          }
        }
        n271 = case shown="3" w154 {
          frame 0, Default {
            n272 = property on="Color Box 43" class="ColBox"("Value"=u32 16711686 ("Color Box")) -> ()  [unwired: 2 in, 2 out]
          }
          frame 1 {
            n273 = property on="Color Box 43" class="ColBox"("Value"=u32 15728450 ("Color Box")) -> ()  [unwired: 2 in, 2 out]
          }
          frame 2 {
            n274 = property on="Color Box 43" class="ColBox"("Value"=u32 16752640 ("Color Box")) -> ()  [unwired: 2 in, 2 out]
          }
          frame 3 {
            n275 = property on="Color Box 43" class="ColBox"("Value"=u32 16711422 ("Color Box")) -> ()  [unwired: 2 in, 2 out]
          }
          frame 4 {
            n276 = property on="Color Box 43" class="ColBox"("Value"=u32 1535 ("Color Box")) -> ()  [unwired: 2 in, 2 out]
          }
          frame 5 {
            n277 = property on="Color Box 43" class="ColBox"("Value"=u32 2621184 ("Color Box")) -> ()  [unwired: 2 in, 2 out]
          }
        }
        n278 = case shown="3" w156 {
          frame 0, Default {
            n279 = property on="Color Box 44" class="ColBox"("Value"=u32 16711686 ("Color Box")) -> ()  [unwired: 2 in, 2 out]
          }
          frame 1 {
            n280 = property on="Color Box 44" class="ColBox"("Value"=u32 15728450 ("Color Box")) -> ()  [unwired: 2 in, 2 out]
          }
          frame 2 {
            n281 = property on="Color Box 44" class="ColBox"("Value"=u32 16752640 ("Color Box")) -> ()  [unwired: 2 in, 2 out]
          }
          frame 3 {
            n282 = property on="Color Box 44" class="ColBox"("Value"=u32 16711422 ("Color Box")) -> ()  [unwired: 2 in, 2 out]
          }
          frame 4 {
            n283 = property on="Color Box 44" class="ColBox"("Value"=u32 1535 ("Color Box")) -> ()  [unwired: 2 in, 2 out]
          }
          frame 5 {
            n284 = property on="Color Box 44" class="ColBox"("Value"=u32 2621184 ("Color Box")) -> ()  [unwired: 2 in, 2 out]
          }
        }
        n285 = case shown="5" w227 {
          frame 0, Default {
            n286 = property on="Color Box 26" class="ColBox"("Value"=u32 16711686 ("Color Box")) -> ()  [unwired: 2 in, 2 out]
          }
          frame 1 {
            n287 = property on="Color Box 26" class="ColBox"("Value"=u32 15728450 ("Color Box")) -> ()  [unwired: 2 in, 2 out]
          }
          frame 2 {
            n288 = property on="Color Box 26" class="ColBox"("Value"=u32 16752640 ("Color Box")) -> ()  [unwired: 2 in, 2 out]
          }
          frame 3 {
            n289 = property on="Color Box 26" class="ColBox"("Value"=u32 16711422 ("Color Box")) -> ()  [unwired: 2 in, 2 out]
          }
          frame 4 {
            n290 = property on="Color Box 26" class="ColBox"("Value"=u32 1535 ("Color Box")) -> ()  [unwired: 2 in, 2 out]
          }
          frame 5 {
            n291 = property on="Color Box 26" class="ColBox"("Value"=u32 2621184 ("Color Box")) -> ()  [unwired: 2 in, 2 out]
          }
        }
        n292 = case shown="3" w225 {
          frame 0, Default {
            n293 = property on="Color Box 25" class="ColBox"("Value"=u32 16711686 ("Color Box")) -> ()  [unwired: 2 in, 2 out]
          }
          frame 1 {
            n294 = property on="Color Box 25" class="ColBox"("Value"=u32 15728450 ("Color Box")) -> ()  [unwired: 2 in, 2 out]
          }
          frame 2 {
            n295 = property on="Color Box 25" class="ColBox"("Value"=u32 16752640 ("Color Box")) -> ()  [unwired: 2 in, 2 out]
          }
          frame 3 {
            n296 = property on="Color Box 25" class="ColBox"("Value"=u32 16711422 ("Color Box")) -> ()  [unwired: 2 in, 2 out]
          }
          frame 4 {
            n297 = property on="Color Box 25" class="ColBox"("Value"=u32 1535 ("Color Box")) -> ()  [unwired: 2 in, 2 out]
          }
          frame 5 {
            n298 = property on="Color Box 25" class="ColBox"("Value"=u32 2621184 ("Color Box")) -> ()  [unwired: 2 in, 2 out]
          }
        }
        n299 = case shown="3" w218 {
          frame 0, Default {
            n300 = property on="Color Box 34" class="ColBox"("Value"=u32 16711686 ("Color Box")) -> ()  [unwired: 2 in, 2 out]
          }
          frame 1 {
            n301 = property on="Color Box 34" class="ColBox"("Value"=u32 15728450 ("Color Box")) -> ()  [unwired: 2 in, 2 out]
          }
          frame 2 {
            n302 = property on="Color Box 34" class="ColBox"("Value"=u32 16752640 ("Color Box")) -> ()  [unwired: 2 in, 2 out]
          }
          frame 3 {
            n303 = property on="Color Box 34" class="ColBox"("Value"=u32 16711422 ("Color Box")) -> ()  [unwired: 2 in, 2 out]
          }
          frame 4 {
            n304 = property on="Color Box 34" class="ColBox"("Value"=u32 1535 ("Color Box")) -> ()  [unwired: 2 in, 2 out]
          }
          frame 5 {
            n305 = property on="Color Box 34" class="ColBox"("Value"=u32 2621184 ("Color Box")) -> ()  [unwired: 2 in, 2 out]
          }
        }
        n306 = case shown="3" w220 {
          frame 0, Default {
            n307 = property on="Color Box 33" class="ColBox"("Value"=u32 16711686 ("Color Box")) -> ()  [unwired: 2 in, 2 out]
          }
          frame 1 {
            n308 = property on="Color Box 33" class="ColBox"("Value"=u32 15728450 ("Color Box")) -> ()  [unwired: 2 in, 2 out]
          }
          frame 2 {
            n309 = property on="Color Box 33" class="ColBox"("Value"=u32 16752640 ("Color Box")) -> ()  [unwired: 2 in, 2 out]
          }
          frame 3 {
            n310 = property on="Color Box 33" class="ColBox"("Value"=u32 16711422 ("Color Box")) -> ()  [unwired: 2 in, 2 out]
          }
          frame 4 {
            n311 = property on="Color Box 33" class="ColBox"("Value"=u32 1535 ("Color Box")) -> ()  [unwired: 2 in, 2 out]
          }
          frame 5 {
            n312 = property on="Color Box 33" class="ColBox"("Value"=u32 2621184 ("Color Box")) -> ()  [unwired: 2 in, 2 out]
          }
        }
        n313 = case shown="3" w131 {
          frame 0, Default {
            n314 = property on="Color Box 47" class="ColBox"("Value"=u32 16711686 ("Color Box")) -> ()  [unwired: 2 in, 2 out]
          }
          frame 1 {
            n315 = property on="Color Box 47" class="ColBox"("Value"=u32 15728450 ("Color Box")) -> ()  [unwired: 2 in, 2 out]
          }
          frame 2 {
            n316 = property on="Color Box 47" class="ColBox"("Value"=u32 16752640 ("Color Box")) -> ()  [unwired: 2 in, 2 out]
          }
          frame 3 {
            n317 = property on="Color Box 47" class="ColBox"("Value"=u32 16711422 ("Color Box")) -> ()  [unwired: 2 in, 2 out]
          }
          frame 4 {
            n318 = property on="Color Box 47" class="ColBox"("Value"=u32 1535 ("Color Box")) -> ()  [unwired: 2 in, 2 out]
          }
          frame 5 {
            n319 = property on="Color Box 47" class="ColBox"("Value"=u32 2621184 ("Color Box")) -> ()  [unwired: 2 in, 2 out]
          }
        }
        n320 = case shown="3" w129 {
          frame 0, Default {
            n321 = property on="Color Box 48" class="ColBox"("Value"=u32 16711686 ("Color Box")) -> ()  [unwired: 2 in, 2 out]
          }
          frame 1 {
            n322 = property on="Color Box 48" class="ColBox"("Value"=u32 15728450 ("Color Box")) -> ()  [unwired: 2 in, 2 out]
          }
          frame 2 {
            n323 = property on="Color Box 48" class="ColBox"("Value"=u32 16752640 ("Color Box")) -> ()  [unwired: 2 in, 2 out]
          }
          frame 3 {
            n324 = property on="Color Box 48" class="ColBox"("Value"=u32 16711422 ("Color Box")) -> ()  [unwired: 2 in, 2 out]
          }
          frame 4 {
            n325 = property on="Color Box 48" class="ColBox"("Value"=u32 1535 ("Color Box")) -> ()  [unwired: 2 in, 2 out]
          }
          frame 5 {
            n326 = property on="Color Box 48" class="ColBox"("Value"=u32 2621184 ("Color Box")) -> ()  [unwired: 2 in, 2 out]
          }
        }
        n327 = case shown="3" w339 {
          frame 0, Default {
            n328 = property on="Color Box 9" class="ColBox"("Value"=u32 16711686 ("Color Box")) -> ()  [unwired: 2 in, 2 out]
          }
          frame 1 {
            n329 = property on="Color Box 9" class="ColBox"("Value"=u32 15728450 ("Color Box")) -> ()  [unwired: 2 in, 2 out]
          }
          frame 2 {
            n330 = property on="Color Box 9" class="ColBox"("Value"=u32 16752640 ("Color Box")) -> ()  [unwired: 2 in, 2 out]
          }
          frame 3 {
            n331 = property on="Color Box 9" class="ColBox"("Value"=u32 16711422 ("Color Box")) -> ()  [unwired: 2 in, 2 out]
          }
          frame 4 {
            n332 = property on="Color Box 9" class="ColBox"("Value"=u32 1535 ("Color Box")) -> ()  [unwired: 2 in, 2 out]
          }
          frame 5 {
            n333 = property on="Color Box 9" class="ColBox"("Value"=u32 2621184 ("Color Box")) -> ()  [unwired: 2 in, 2 out]
          }
        }
        n334 = case shown="3" w337 {
          frame 0, Default {
            n335 = property on="Color Box 10" class="ColBox"("Value"=u32 16711686 ("Color Box")) -> ()  [unwired: 2 in, 2 out]
          }
          frame 1 {
            n336 = property on="Color Box 10" class="ColBox"("Value"=u32 15728450 ("Color Box")) -> ()  [unwired: 2 in, 2 out]
          }
          frame 2 {
            n337 = property on="Color Box 10" class="ColBox"("Value"=u32 16752640 ("Color Box")) -> ()  [unwired: 2 in, 2 out]
          }
          frame 3 {
            n338 = property on="Color Box 10" class="ColBox"("Value"=u32 16711422 ("Color Box")) -> ()  [unwired: 2 in, 2 out]
          }
          frame 4 {
            n339 = property on="Color Box 10" class="ColBox"("Value"=u32 1535 ("Color Box")) -> ()  [unwired: 2 in, 2 out]
          }
          frame 5 {
            n340 = property on="Color Box 10" class="ColBox"("Value"=u32 2621184 ("Color Box")) -> ()  [unwired: 2 in, 2 out]
          }
        }
        n341 = case shown="3" w282 {
          frame 0, Default {
            n342 = property on="Color Box 17" class="ColBox"("Value"=u32 16711686 ("Color Box")) -> ()  [unwired: 2 in, 2 out]
          }
          frame 1 {
            n343 = property on="Color Box 17" class="ColBox"("Value"=u32 15728450 ("Color Box")) -> ()  [unwired: 2 in, 2 out]
          }
          frame 2 {
            n344 = property on="Color Box 17" class="ColBox"("Value"=u32 16752640 ("Color Box")) -> ()  [unwired: 2 in, 2 out]
          }
          frame 3 {
            n345 = property on="Color Box 17" class="ColBox"("Value"=u32 16711422 ("Color Box")) -> ()  [unwired: 2 in, 2 out]
          }
          frame 4 {
            n346 = property on="Color Box 17" class="ColBox"("Value"=u32 1535 ("Color Box")) -> ()  [unwired: 2 in, 2 out]
          }
          frame 5 {
            n347 = property on="Color Box 17" class="ColBox"("Value"=u32 2621184 ("Color Box")) -> ()  [unwired: 2 in, 2 out]
          }
        }
        n348 = case shown="3" w284 {
          frame 0, Default {
            n349 = property on="Color Box 18" class="ColBox"("Value"=u32 16711686 ("Color Box")) -> ()  [unwired: 2 in, 2 out]
          }
          frame 1 {
            n350 = property on="Color Box 18" class="ColBox"("Value"=u32 15728450 ("Color Box")) -> ()  [unwired: 2 in, 2 out]
          }
          frame 2 {
            n351 = property on="Color Box 18" class="ColBox"("Value"=u32 16752640 ("Color Box")) -> ()  [unwired: 2 in, 2 out]
          }
          frame 3 {
            n352 = property on="Color Box 18" class="ColBox"("Value"=u32 16711422 ("Color Box")) -> ()  [unwired: 2 in, 2 out]
          }
          frame 4 {
            n353 = property on="Color Box 18" class="ColBox"("Value"=u32 1535 ("Color Box")) -> ()  [unwired: 2 in, 2 out]
          }
          frame 5 {
            n354 = property on="Color Box 18" class="ColBox"("Value"=u32 2621184 ("Color Box")) -> ()  [unwired: 2 in, 2 out]
          }
        }
        n355 = case shown="3" w330 {
          frame 0, Default {
            n356 = property on="Color Box 13" class="ColBox"("Value"=u32 16711686 ("Color Box")) -> ()  [unwired: 2 in, 2 out]
          }
          frame 1 {
            n357 = property on="Color Box 13" class="ColBox"("Value"=u32 15728450 ("Color Box")) -> ()  [unwired: 2 in, 2 out]
          }
          frame 2 {
            n358 = property on="Color Box 13" class="ColBox"("Value"=u32 16752640 ("Color Box")) -> ()  [unwired: 2 in, 2 out]
          }
          frame 3 {
            n359 = property on="Color Box 13" class="ColBox"("Value"=u32 16711422 ("Color Box")) -> ()  [unwired: 2 in, 2 out]
          }
          frame 4 {
            n360 = property on="Color Box 13" class="ColBox"("Value"=u32 1535 ("Color Box")) -> ()  [unwired: 2 in, 2 out]
          }
          frame 5 {
            n361 = property on="Color Box 13" class="ColBox"("Value"=u32 2621184 ("Color Box")) -> ()  [unwired: 2 in, 2 out]
          }
        }
        n362 = case shown="3" w332 {
          frame 0, Default {
            n363 = property on="Color Box 14" class="ColBox"("Value"=u32 16711686 ("Color Box")) -> ()  [unwired: 2 in, 2 out]
          }
          frame 1 {
            n364 = property on="Color Box 14" class="ColBox"("Value"=u32 15728450 ("Color Box")) -> ()  [unwired: 2 in, 2 out]
          }
          frame 2 {
            n365 = property on="Color Box 14" class="ColBox"("Value"=u32 16752640 ("Color Box")) -> ()  [unwired: 2 in, 2 out]
          }
          frame 3 {
            n366 = property on="Color Box 14" class="ColBox"("Value"=u32 16711422 ("Color Box")) -> ()  [unwired: 2 in, 2 out]
          }
          frame 4 {
            n367 = property on="Color Box 14" class="ColBox"("Value"=u32 1535 ("Color Box")) -> ()  [unwired: 2 in, 2 out]
          }
          frame 5 {
            n368 = property on="Color Box 14" class="ColBox"("Value"=u32 2621184 ("Color Box")) -> ()  [unwired: 2 in, 2 out]
          }
        }
        n369 = case shown="3" w291 {
          frame 0, Default {
            n370 = property on="Color Box 21" class="ColBox"("Value"=u32 16711686 ("Color Box")) -> ()  [unwired: 2 in, 2 out]
          }
          frame 1 {
            n371 = property on="Color Box 21" class="ColBox"("Value"=u32 15728450 ("Color Box")) -> ()  [unwired: 2 in, 2 out]
          }
          frame 2 {
            n372 = property on="Color Box 21" class="ColBox"("Value"=u32 16752640 ("Color Box")) -> ()  [unwired: 2 in, 2 out]
          }
          frame 3 {
            n373 = property on="Color Box 21" class="ColBox"("Value"=u32 16711422 ("Color Box")) -> ()  [unwired: 2 in, 2 out]
          }
          frame 4 {
            n374 = property on="Color Box 21" class="ColBox"("Value"=u32 1535 ("Color Box")) -> ()  [unwired: 2 in, 2 out]
          }
          frame 5 {
            n375 = property on="Color Box 21" class="ColBox"("Value"=u32 2621184 ("Color Box")) -> ()  [unwired: 2 in, 2 out]
          }
        }
        n376 = case shown="3" w289 {
          frame 0, Default {
            n377 = property on="Color Box 22" class="ColBox"("Value"=u32 16711686 ("Color Box")) -> ()  [unwired: 2 in, 2 out]
          }
          frame 1 {
            n378 = property on="Color Box 22" class="ColBox"("Value"=u32 15728450 ("Color Box")) -> ()  [unwired: 2 in, 2 out]
          }
          frame 2 {
            n379 = property on="Color Box 22" class="ColBox"("Value"=u32 16752640 ("Color Box")) -> ()  [unwired: 2 in, 2 out]
          }
          frame 3 {
            n380 = property on="Color Box 22" class="ColBox"("Value"=u32 16711422 ("Color Box")) -> ()  [unwired: 2 in, 2 out]
          }
          frame 4 {
            n381 = property on="Color Box 22" class="ColBox"("Value"=u32 1535 ("Color Box")) -> ()  [unwired: 2 in, 2 out]
          }
          frame 5 {
            n382 = property on="Color Box 22" class="ColBox"("Value"=u32 2621184 ("Color Box")) -> ()  [unwired: 2 in, 2 out]
          }
        }
        n383 = case shown="3" w346 {
          frame 0, Default {
            n384 = property on="Color Box 11" class="ColBox"("Value"=u32 16711686 ("Color Box")) -> ()  [unwired: 2 in, 2 out]
          }
          frame 1 {
            n385 = property on="Color Box 11" class="ColBox"("Value"=u32 15728450 ("Color Box")) -> ()  [unwired: 2 in, 2 out]
          }
          frame 2 {
            n386 = property on="Color Box 11" class="ColBox"("Value"=u32 16752640 ("Color Box")) -> ()  [unwired: 2 in, 2 out]
          }
          frame 3 {
            n387 = property on="Color Box 11" class="ColBox"("Value"=u32 16711422 ("Color Box")) -> ()  [unwired: 2 in, 2 out]
          }
          frame 4 {
            n388 = property on="Color Box 11" class="ColBox"("Value"=u32 1535 ("Color Box")) -> ()  [unwired: 2 in, 2 out]
          }
          frame 5 {
            n389 = property on="Color Box 11" class="ColBox"("Value"=u32 2621184 ("Color Box")) -> ()  [unwired: 2 in, 2 out]
          }
        }
        n390 = case shown="3" w348 {
          frame 0, Default {
            n391 = property on="Color Box 12" class="ColBox"("Value"=u32 16711686 ("Color Box")) -> ()  [unwired: 2 in, 2 out]
          }
          frame 1 {
            n392 = property on="Color Box 12" class="ColBox"("Value"=u32 15728450 ("Color Box")) -> ()  [unwired: 2 in, 2 out]
          }
          frame 2 {
            n393 = property on="Color Box 12" class="ColBox"("Value"=u32 16752640 ("Color Box")) -> ()  [unwired: 2 in, 2 out]
          }
          frame 3 {
            n394 = property on="Color Box 12" class="ColBox"("Value"=u32 16711422 ("Color Box")) -> ()  [unwired: 2 in, 2 out]
          }
          frame 4 {
            n395 = property on="Color Box 12" class="ColBox"("Value"=u32 1535 ("Color Box")) -> ()  [unwired: 2 in, 2 out]
          }
          frame 5 {
            n396 = property on="Color Box 12" class="ColBox"("Value"=u32 2621184 ("Color Box")) -> ()  [unwired: 2 in, 2 out]
          }
        }
        n397 = case shown="3" w275 {
          frame 0, Default {
            n398 = property on="Color Box 19" class="ColBox"("Value"=u32 16711686 ("Color Box")) -> ()  [unwired: 2 in, 2 out]
          }
          frame 1 {
            n399 = property on="Color Box 19" class="ColBox"("Value"=u32 15728450 ("Color Box")) -> ()  [unwired: 2 in, 2 out]
          }
          frame 2 {
            n400 = property on="Color Box 19" class="ColBox"("Value"=u32 16752640 ("Color Box")) -> ()  [unwired: 2 in, 2 out]
          }
          frame 3 {
            n401 = property on="Color Box 19" class="ColBox"("Value"=u32 16711422 ("Color Box")) -> ()  [unwired: 2 in, 2 out]
          }
          frame 4 {
            n402 = property on="Color Box 19" class="ColBox"("Value"=u32 1535 ("Color Box")) -> ()  [unwired: 2 in, 2 out]
          }
          frame 5 {
            n403 = property on="Color Box 19" class="ColBox"("Value"=u32 2621184 ("Color Box")) -> ()  [unwired: 2 in, 2 out]
          }
        }
        n404 = case shown="3" w273 {
          frame 0, Default {
            n405 = property on="Color Box 20" class="ColBox"("Value"=u32 16711686 ("Color Box")) -> ()  [unwired: 2 in, 2 out]
          }
          frame 1 {
            n406 = property on="Color Box 20" class="ColBox"("Value"=u32 15728450 ("Color Box")) -> ()  [unwired: 2 in, 2 out]
          }
          frame 2 {
            n407 = property on="Color Box 20" class="ColBox"("Value"=u32 16752640 ("Color Box")) -> ()  [unwired: 2 in, 2 out]
          }
          frame 3 {
            n408 = property on="Color Box 20" class="ColBox"("Value"=u32 16711422 ("Color Box")) -> ()  [unwired: 2 in, 2 out]
          }
          frame 4 {
            n409 = property on="Color Box 20" class="ColBox"("Value"=u32 1535 ("Color Box")) -> ()  [unwired: 2 in, 2 out]
          }
          frame 5 {
            n410 = property on="Color Box 20" class="ColBox"("Value"=u32 2621184 ("Color Box")) -> ()  [unwired: 2 in, 2 out]
          }
        }
        n411 = case shown="3" w370 {
          frame 0, Default {
            n412 = property on="Color Box 5" class="ColBox"("Value"=u32 16711686 ("Color Box")) -> ()  [unwired: 2 in, 2 out]
          }
          frame 1 {
            n413 = property on="Color Box 5" class="ColBox"("Value"=u32 15728450 ("Color Box")) -> ()  [unwired: 2 in, 2 out]
          }
          frame 2 {
            n414 = property on="Color Box 5" class="ColBox"("Value"=u32 16752640 ("Color Box")) -> ()  [unwired: 2 in, 2 out]
          }
          frame 3 {
            n415 = property on="Color Box 5" class="ColBox"("Value"=u32 16711422 ("Color Box")) -> ()  [unwired: 2 in, 2 out]
          }
          frame 4 {
            n416 = property on="Color Box 5" class="ColBox"("Value"=u32 1535 ("Color Box")) -> ()  [unwired: 2 in, 2 out]
          }
          frame 5 {
            n417 = property on="Color Box 5" class="ColBox"("Value"=u32 2621184 ("Color Box")) -> ()  [unwired: 2 in, 2 out]
          }
        }
        n418 = case shown="3" w372 {
          frame 0, Default {
            n419 = property on="Color Box 6" class="ColBox"("Value"=u32 16711686 ("Color Box")) -> ()  [unwired: 2 in, 2 out]
          }
          frame 1 {
            n420 = property on="Color Box 6" class="ColBox"("Value"=u32 15728450 ("Color Box")) -> ()  [unwired: 2 in, 2 out]
          }
          frame 2 {
            n421 = property on="Color Box 6" class="ColBox"("Value"=u32 16752640 ("Color Box")) -> ()  [unwired: 2 in, 2 out]
          }
          frame 3 {
            n422 = property on="Color Box 6" class="ColBox"("Value"=u32 16711422 ("Color Box")) -> ()  [unwired: 2 in, 2 out]
          }
          frame 4 {
            n423 = property on="Color Box 6" class="ColBox"("Value"=u32 1535 ("Color Box")) -> ()  [unwired: 2 in, 2 out]
          }
          frame 5 {
            n424 = property on="Color Box 6" class="ColBox"("Value"=u32 2621184 ("Color Box")) -> ()  [unwired: 2 in, 2 out]
          }
        }
        n425 = case shown="2" w323 {
          frame 0, Default {
            n426 = property on="Color Box 15" class="ColBox"("Value"=u32 16711686 ("Color Box")) -> ()  [unwired: 2 in, 2 out]
          }
          frame 1 {
            n427 = property on="Color Box 15" class="ColBox"("Value"=u32 15728450 ("Color Box")) -> ()  [unwired: 2 in, 2 out]
          }
          frame 2 {
            n428 = property on="Color Box 15" class="ColBox"("Value"=u32 16752640 ("Color Box")) -> ()  [unwired: 2 in, 2 out]
          }
          frame 3 {
            n429 = property on="Color Box 15" class="ColBox"("Value"=u32 16711422 ("Color Box")) -> ()  [unwired: 2 in, 2 out]
          }
          frame 4 {
            n430 = property on="Color Box 15" class="ColBox"("Value"=u32 1535 ("Color Box")) -> ()  [unwired: 2 in, 2 out]
          }
          frame 5 {
            n431 = property on="Color Box 15" class="ColBox"("Value"=u32 2621184 ("Color Box")) -> ()  [unwired: 2 in, 2 out]
          }
        }
        n432 = case shown="3" w321 {
          frame 0, Default {
            n433 = property on="Color Box 16" class="ColBox"("Value"=u32 16711686 ("Color Box")) -> ()  [unwired: 2 in, 2 out]
          }
          frame 1 {
            n434 = property on="Color Box 16" class="ColBox"("Value"=u32 15728450 ("Color Box")) -> ()  [unwired: 2 in, 2 out]
          }
          frame 2 {
            n435 = property on="Color Box 16" class="ColBox"("Value"=u32 16752640 ("Color Box")) -> ()  [unwired: 2 in, 2 out]
          }
          frame 3 {
            n436 = property on="Color Box 16" class="ColBox"("Value"=u32 16711422 ("Color Box")) -> ()  [unwired: 2 in, 2 out]
          }
          frame 4 {
            n437 = property on="Color Box 16" class="ColBox"("Value"=u32 1535 ("Color Box")) -> ()  [unwired: 2 in, 2 out]
          }
          frame 5 {
            n438 = property on="Color Box 16" class="ColBox"("Value"=u32 2621184 ("Color Box")) -> ()  [unwired: 2 in, 2 out]
          }
        }
        n439 = case shown="1" w298 {
          frame 0, Default {
            n440 = property on="Color Box 23" class="ColBox"("Value"=u32 16711686 ("Color Box")) -> ()  [unwired: 2 in, 2 out]
          }
          frame 1 {
            n441 = property on="Color Box 23" class="ColBox"("Value"=u32 15728450 ("Color Box")) -> ()  [unwired: 2 in, 2 out]
          }
          frame 2 {
            n442 = property on="Color Box 23" class="ColBox"("Value"=u32 16752640 ("Color Box")) -> ()  [unwired: 2 in, 2 out]
          }
          frame 3 {
            n443 = property on="Color Box 23" class="ColBox"("Value"=u32 16711422 ("Color Box")) -> ()  [unwired: 2 in, 2 out]
          }
          frame 4 {
            n444 = property on="Color Box 23" class="ColBox"("Value"=u32 1535 ("Color Box")) -> ()  [unwired: 2 in, 2 out]
          }
          frame 5 {
            n445 = property on="Color Box 23" class="ColBox"("Value"=u32 2621184 ("Color Box")) -> ()  [unwired: 2 in, 2 out]
          }
        }
        n446 = case shown="3" w300 {
          frame 0, Default {
            n447 = property on="Color Box 24" class="ColBox"("Value"=u32 16711686 ("Color Box")) -> ()  [unwired: 2 in, 2 out]
          }
          frame 1 {
            n448 = property on="Color Box 24" class="ColBox"("Value"=u32 15728450 ("Color Box")) -> ()  [unwired: 2 in, 2 out]
          }
          frame 2 {
            n449 = property on="Color Box 24" class="ColBox"("Value"=u32 16752640 ("Color Box")) -> ()  [unwired: 2 in, 2 out]
          }
          frame 3 {
            n450 = property on="Color Box 24" class="ColBox"("Value"=u32 16711422 ("Color Box")) -> ()  [unwired: 2 in, 2 out]
          }
          frame 4 {
            n451 = property on="Color Box 24" class="ColBox"("Value"=u32 1535 ("Color Box")) -> ()  [unwired: 2 in, 2 out]
          }
          frame 5 {
            n452 = property on="Color Box 24" class="ColBox"("Value"=u32 2621184 ("Color Box")) -> ()  [unwired: 2 in, 2 out]
          }
        }
        n453 = case shown="3" w383 {
          frame 0, Default {
            n454 = property on="Color Box 3" class="ColBox"("Value"=u32 16711686 ("Color Box")) -> ()  [unwired: 2 in, 2 out]
          }
          frame 1 {
            n455 = property on="Color Box 3" class="ColBox"("Value"=u32 15728450 ("Color Box")) -> ()  [unwired: 2 in, 2 out]
          }
          frame 2 {
            n456 = property on="Color Box 3" class="ColBox"("Value"=u32 16752640 ("Color Box")) -> ()  [unwired: 2 in, 2 out]
          }
          frame 3 {
            n457 = property on="Color Box 3" class="ColBox"("Value"=u32 16711422 ("Color Box")) -> ()  [unwired: 2 in, 2 out]
          }
          frame 4 {
            n458 = property on="Color Box 3" class="ColBox"("Value"=u32 1535 ("Color Box")) -> ()  [unwired: 2 in, 2 out]
          }
          frame 5 {
            n459 = property on="Color Box 3" class="ColBox"("Value"=u32 2621184 ("Color Box")) -> ()  [unwired: 2 in, 2 out]
          }
        }
        n460 = case shown="3" w381 {
          frame 0, Default {
            n461 = property on="Color Box 4" class="ColBox"("Value"=u32 16711686 ("Color Box")) -> ()  [unwired: 2 in, 2 out]
          }
          frame 1 {
            n462 = property on="Color Box 4" class="ColBox"("Value"=u32 15728450 ("Color Box")) -> ()  [unwired: 2 in, 2 out]
          }
          frame 2 {
            n463 = property on="Color Box 4" class="ColBox"("Value"=u32 16752640 ("Color Box")) -> ()  [unwired: 2 in, 2 out]
          }
          frame 3 {
            n464 = property on="Color Box 4" class="ColBox"("Value"=u32 16711422 ("Color Box")) -> ()  [unwired: 2 in, 2 out]
          }
          frame 4 {
            n465 = property on="Color Box 4" class="ColBox"("Value"=u32 1535 ("Color Box")) -> ()  [unwired: 2 in, 2 out]
          }
          frame 5 {
            n466 = property on="Color Box 4" class="ColBox"("Value"=u32 2621184 ("Color Box")) -> ()  [unwired: 2 in, 2 out]
          }
        }
        n467 = case shown="3" w363 {
          frame 0, Default {
            n468 = property on="Color Box 7" class="ColBox"("Value"=u32 16711686 ("Color Box")) -> ()  [unwired: 2 in, 2 out]
          }
          frame 1 {
            n469 = property on="Color Box 7" class="ColBox"("Value"=u32 15728450 ("Color Box")) -> ()  [unwired: 2 in, 2 out]
          }
          frame 2 {
            n470 = property on="Color Box 7" class="ColBox"("Value"=u32 16752640 ("Color Box")) -> ()  [unwired: 2 in, 2 out]
          }
          frame 3 {
            n471 = property on="Color Box 7" class="ColBox"("Value"=u32 16711422 ("Color Box")) -> ()  [unwired: 2 in, 2 out]
          }
          frame 4 {
            n472 = property on="Color Box 7" class="ColBox"("Value"=u32 1535 ("Color Box")) -> ()  [unwired: 2 in, 2 out]
          }
          frame 5 {
            n473 = property on="Color Box 7" class="ColBox"("Value"=u32 2621184 ("Color Box")) -> ()  [unwired: 2 in, 2 out]
          }
        }
        n474 = case shown="3" w361 {
          frame 0, Default {
            n475 = property on="Color Box 8" class="ColBox"("Value"=u32 16711686 ("Color Box")) -> ()  [unwired: 2 in, 2 out]
          }
          frame 1 {
            n476 = property on="Color Box 8" class="ColBox"("Value"=u32 15728450 ("Color Box")) -> ()  [unwired: 2 in, 2 out]
          }
          frame 2 {
            n477 = property on="Color Box 8" class="ColBox"("Value"=u32 16752640 ("Color Box")) -> ()  [unwired: 2 in, 2 out]
          }
          frame 3 {
            n478 = property on="Color Box 8" class="ColBox"("Value"=u32 16711422 ("Color Box")) -> ()  [unwired: 2 in, 2 out]
          }
          frame 4 {
            n479 = property on="Color Box 8" class="ColBox"("Value"=u32 1535 ("Color Box")) -> ()  [unwired: 2 in, 2 out]
          }
          frame 5 {
            n480 = property on="Color Box 8" class="ColBox"("Value"=u32 2621184 ("Color Box")) -> ()  [unwired: 2 in, 2 out]
          }
        }
        n481 = case shown="0, Default" w393 {
          frame 0, Default {
            n482 = property on="Color Box 2" class="ColBox"("Value"=u32 16711686 ("Color Box")) -> ()  [unwired: 2 in, 2 out]
          }
          frame 1 {
            n483 = property on="Color Box 2" class="ColBox"("Value"=u32 15728450 ("Color Box")) -> ()  [unwired: 2 in, 2 out]
          }
          frame 2 {
            n484 = property on="Color Box 2" class="ColBox"("Value"=u32 16752640 ("Color Box")) -> ()  [unwired: 2 in, 2 out]
          }
          frame 3 {
            n485 = property on="Color Box 2" class="ColBox"("Value"=u32 16711422 ("Color Box")) -> ()  [unwired: 2 in, 2 out]
          }
          frame 4 {
            n486 = property on="Color Box 2" class="ColBox"("Value"=u32 1535 ("Color Box")) -> ()  [unwired: 2 in, 2 out]
          }
          frame 5 {
            n487 = property on="Color Box 2" class="ColBox"("Value"=u32 2621184 ("Color Box")) -> ()  [unwired: 2 in, 2 out]
          }
        }
        n488 = case shown="3" w395 {
          frame 0, Default {
            n489 = property on="Color Box" class="ColBox"("Value"=u32 16711686 ("Color Box")) -> ()  [unwired: 2 in, 2 out]
          }
          frame 1 {
            n490 = property on="Color Box" class="ColBox"("Value"=u32 15728450 ("Color Box")) -> ()  [unwired: 2 in, 2 out]
          }
          frame 2 {
            n491 = property on="Color Box" class="ColBox"("Value"=u32 16752640 ("Color Box")) -> ()  [unwired: 2 in, 2 out]
          }
          frame 3 {
            n492 = property on="Color Box" class="ColBox"("Value"=u32 16711422 ("Color Box")) -> ()  [unwired: 2 in, 2 out]
          }
          frame 4 {
            n493 = property on="Color Box" class="ColBox"("Value"=u32 1535 ("Color Box")) -> ()  [unwired: 2 in, 2 out]
          }
          frame 5 {
            n494 = property on="Color Box" class="ColBox"("Value"=u32 2621184 ("Color Box")) -> ()  [unwired: 2 in, 2 out]
          }
        }
      }
      n495 = disable-structure shown="Disabled" {
        frame Disabled {
          n496 = property on="Blanc" class="DigNum (strict)" props=["Value"]() -> ()  [unwired: 2 in, 3 out]
          n497 = property on="Jaune" class="DigNum (strict)" props=["Value"]() -> ()  [unwired: 2 in, 3 out]
          n498 = property on="Bleu" class="DigNum (strict)" props=["Value"]() -> ()  [unwired: 2 in, 3 out]
          n499 = property on="Orange" class="DigNum (strict)" props=["Value"]() -> ()  [unwired: 2 in, 3 out]
          n500 = property on="Vert" class="DigNum (strict)" props=["Value"]() -> ()  [unwired: 2 in, 3 out]
        }
        frame Enabled {
        }
      }
    }
    frame #1 {
      n501 = property on="Color Box 12" class="ColBox"() -> ("Value"=w783:u32)  [unwired: 2 in, 2 out]
      n502 = property on="Color Box 16" class="ColBox"() -> ("Value"=w779:u32)  [unwired: 2 in, 2 out]
      n503 = property on="Color Box 13" class="ColBox"() -> ("Value"=w780:u32)  [unwired: 2 in, 2 out]
      n504 = property on="Color Box 14" class="ColBox"() -> ("Value"=w781:u32)  [unwired: 2 in, 2 out]
      n505 = property on="Color Box 11" class="ColBox"() -> ("Value"=w782:u32)  [unwired: 2 in, 2 out]
      n506 = property on="Color Box 10" class="ColBox"() -> ("Value"=w785:u32)  [unwired: 2 in, 2 out]
      n507 = property on="Color Box 15" class="ColBox"() -> ("Value"=w778:u32)  [unwired: 2 in, 2 out]
      n508 = property on="Color Box 9" class="ColBox"() -> ("Value"=w784:u32)  [unwired: 2 in, 2 out]
      n509 = property on="Color Box 2" class="ColBox"() -> ("Value"=w795:u32)  [unwired: 2 in, 2 out]
      n510 = property on="Color Box 6" class="ColBox"() -> ("Value"=w789:u32)  [unwired: 2 in, 2 out]
      n511 = property on="Color Box" class="ColBox"() -> ("Value"=w794:u32)  [unwired: 2 in, 2 out]
      n512 = property on="Color Box 8" class="ColBox"() -> ("Value"=w790:u32)  [unwired: 2 in, 2 out]
      n513 = property on="Color Box 5" class="ColBox"() -> ("Value"=w788:u32)  [unwired: 2 in, 2 out]
      n514 = property on="Color Box 7" class="ColBox"() -> ("Value"=w791:u32)  [unwired: 2 in, 2 out]
      n515 = property on="Color Box 3" class="ColBox"() -> ("Value"=w793:u32)  [unwired: 2 in, 2 out]
      n516 = property on="Color Box 4" class="ColBox"() -> ("Value"=w792:u32)  [unwired: 2 in, 2 out]
      n517 = property on="Color Box 23" class="ColBox"() -> ("Value"=w776:u32)  [unwired: 2 in, 2 out]
      n518 = property on="Color Box 46" class="ColBox"() -> ("Value"=w746:u32)  [unwired: 2 in, 2 out]
      n519 = property on="Color Box 48" class="ColBox"() -> ("Value"=w748:u32)  [unwired: 2 in, 2 out]
      n520 = property on="Color Box 47" class="ColBox"() -> ("Value"=w749:u32)  [unwired: 2 in, 2 out]
      n521 = property on="Color Box 43" class="ColBox"() -> ("Value"=w745:u32)  [unwired: 2 in, 2 out]
      n522 = property on="Color Box 24" class="ColBox"() -> ("Value"=w775:u32)  [unwired: 2 in, 2 out]
      n523 = property on="Color Box 42" class="ColBox"() -> ("Value"=w742:u32)  [unwired: 2 in, 2 out]
      n524 = property on="Color Box 21" class="ColBox"() -> ("Value"=w774:u32)  [unwired: 2 in, 2 out]
      n525 = property on="Color Box 18" class="ColBox"() -> ("Value"=w769:u32)  [unwired: 2 in, 2 out]
      n526 = property on="Color Box 45" class="ColBox"() -> ("Value"=w747:u32)  [unwired: 2 in, 2 out]
      n527 = property on="Color Box 20" class="ColBox"() -> ("Value"=w771:u32)  [unwired: 2 in, 2 out]
      n528 = property on="Color Box 22" class="ColBox"() -> ("Value"=w773:u32)  [unwired: 2 in, 2 out]
      n529 = property on="Color Box 19" class="ColBox"() -> ("Value"=w772:u32)  [unwired: 2 in, 2 out]
      n530 = property on="Color Box 17" class="ColBox"() -> ("Value"=w770:u32)  [unwired: 2 in, 2 out]
      n531 = property on="Color Box 26" class="ColBox"() -> ("Value"=w767:u32)  [unwired: 2 in, 2 out]
      n532 = property on="Color Box 41" class="ColBox"() -> ("Value"=w743:u32)  [unwired: 2 in, 2 out]
      n533 = property on="Color Box 44" class="ColBox"() -> ("Value"=w744:u32)  [unwired: 2 in, 2 out]
      n534 = property on="Color Box 25" class="ColBox"() -> ("Value"=w766:u32)  [unwired: 2 in, 2 out]
      n535 = property on="Color Box 28" class="ColBox"() -> ("Value"=w765:u32)  [unwired: 2 in, 2 out]
      n536 = property on="Color Box 36" class="ColBox"() -> ("Value"=w756:u32)  [unwired: 2 in, 2 out]
      n537 = property on="Color Box 27" class="ColBox"() -> ("Value"=w764:u32)  [unwired: 2 in, 2 out]
      n538 = property on="Color Box 34" class="ColBox"() -> ("Value"=w758:u32)  [unwired: 2 in, 2 out]
      n539 = property on="Color Box 33" class="ColBox"() -> ("Value"=w757:u32)  [unwired: 2 in, 2 out]
      n540 = property on="Color Box 35" class="ColBox"() -> ("Value"=w755:u32)  [unwired: 2 in, 2 out]
      n541 = property on="Color Box 29" class="ColBox"() -> ("Value"=w762:u32)  [unwired: 2 in, 2 out]
      n542 = property on="Color Box 30" class="ColBox"() -> ("Value"=w763:u32)  [unwired: 2 in, 2 out]
      n543 = property on="Color Box 38" class="ColBox"() -> ("Value"=w754:u32)  [unwired: 2 in, 2 out]
      n544 = property on="Color Box 31" class="ColBox"() -> ("Value"=w760:u32)  [unwired: 2 in, 2 out]
      n545 = property on="Color Box 40" class="ColBox"() -> ("Value"=w752:u32)  [unwired: 2 in, 2 out]
      n546 = property on="Color Box 37" class="ColBox"() -> ("Value"=w753:u32)  [unwired: 2 in, 2 out]
      n547 = property on="Color Box 39" class="ColBox"() -> ("Value"=w751:u32)  [unwired: 2 in, 2 out]
      n548 = property on="Color Box 32" class="ColBox"() -> ("Value"=w761:u32)  [unwired: 2 in, 2 out]
      n549 = case shown="2621184" w794 {
        tunnel: [404 1 3 2 0 5 4] -> w741
        frame Default {
        }
        frame 16711686 {
        }
        frame 15728450 {
        }
        frame 16752640 {
        }
        frame 16711422 {
        }
        frame 1535 {
        }
        frame 2621184 {
        }
      }
      n550 = case shown="1535" w795 {
        tunnel: [404 1 3 2 0 5 4] -> w738
        frame Default {
        }
        frame 16711686 {
        }
        frame 15728450 {
        }
        frame 16752640 {
        }
        frame 16711422 {
        }
        frame 1535 {
        }
        frame 2621184 {
        }
      }
      n551 = case shown="2621184" w788 {
        tunnel: [404 1 3 2 0 5 4] -> w735
        frame Default {
        }
        frame 16711686 {
        }
        frame 15728450 {
        }
        frame 16752640 {
        }
        frame 16711422 {
        }
        frame 1535 {
        }
        frame 2621184 {
        }
      }
      n552 = case shown="2621184" w793 {
        tunnel: [404 1 3 2 0 5 4] -> w740
        frame Default {
        }
        frame 16711686 {
        }
        frame 15728450 {
        }
        frame 16752640 {
        }
        frame 16711422 {
        }
        frame 1535 {
        }
        frame 2621184 {
        }
      }
      n553 = case shown="2621184" w792 {
        tunnel: [404 1 3 2 0 5 4] -> w739
        frame Default {
        }
        frame 16711686 {
        }
        frame 15728450 {
        }
        frame 16752640 {
        }
        frame 16711422 {
        }
        frame 1535 {
        }
        frame 2621184 {
        }
      }
      n554 = case shown="2621184" w790 {
        tunnel: [404 1 3 2 0 5 4] -> w736
        frame Default {
        }
        frame 16711686 {
        }
        frame 15728450 {
        }
        frame 16752640 {
        }
        frame 16711422 {
        }
        frame 1535 {
        }
        frame 2621184 {
        }
      }
      n555 = case shown="2621184" w791 {
        tunnel: [404 1 3 2 0 5 4] -> w737
        frame Default {
        }
        frame 16711686 {
        }
        frame 15728450 {
        }
        frame 16752640 {
        }
        frame 16711422 {
        }
        frame 1535 {
        }
        frame 2621184 {
        }
      }
      n556 = case shown="2621184" w789 {
        tunnel: [404 1 3 2 0 5 4] -> w734
        frame Default {
        }
        frame 16711686 {
        }
        frame 15728450 {
        }
        frame 16752640 {
        }
        frame 16711422 {
        }
        frame 1535 {
        }
        frame 2621184 {
        }
      }
      n557 = case shown="2621184" w779 {
        tunnel: [404 1 3 2 0 5 4] -> w732
        frame Default {
        }
        frame 16711686 {
        }
        frame 15728450 {
        }
        frame 16752640 {
        }
        frame 16711422 {
        }
        frame 1535 {
        }
        frame 2621184 {
        }
      }
      n558 = case shown="1535" w778 {
        tunnel: [404 1 3 2 0 5 4] -> w733
        frame Default {
        }
        frame 16711686 {
        }
        frame 15728450 {
        }
        frame 16752640 {
        }
        frame 16711422 {
        }
        frame 1535 {
        }
        frame 2621184 {
        }
      }
      n559 = case shown="2621184" w784 {
        tunnel: [404 1 3 2 0 5 4] -> w727
        frame Default {
        }
        frame 16711686 {
        }
        frame 15728450 {
        }
        frame 16752640 {
        }
        frame 16711422 {
        }
        frame 1535 {
        }
        frame 2621184 {
        }
      }
      n560 = case shown="2621184" w780 {
        tunnel: [404 1 3 2 0 5 4] -> w731
        frame Default {
        }
        frame 16711686 {
        }
        frame 15728450 {
        }
        frame 16752640 {
        }
        frame 16711422 {
        }
        frame 1535 {
        }
        frame 2621184 {
        }
      }
      n561 = case shown="2621184" w781 {
        tunnel: [404 1 3 2 0 5 4] -> w730
        frame Default {
        }
        frame 16711686 {
        }
        frame 15728450 {
        }
        frame 16752640 {
        }
        frame 16711422 {
        }
        frame 1535 {
        }
        frame 2621184 {
        }
      }
      n562 = case shown="2621184" w775 {
        tunnel: [404 1 3 2 0 5 4] -> w724
        frame Default {
        }
        frame 16711686 {
        }
        frame 15728450 {
        }
        frame 16752640 {
        }
        frame 16711422 {
        }
        frame 1535 {
        }
        frame 2621184 {
        }
      }
      n563 = case shown="1535" w776 {
        tunnel: [404 1 3 2 0 5 4] -> w725
        frame Default {
        }
        frame 16711686 {
        }
        frame 15728450 {
        }
        frame 16752640 {
        }
        frame 16711422 {
        }
        frame 1535 {
        }
        frame 2621184 {
        }
      }
      n564 = case shown="2621184" w783 {
        tunnel: [404 1 3 2 0 5 4] -> w728
        frame Default {
        }
        frame 16711686 {
        }
        frame 15728450 {
        }
        frame 16752640 {
        }
        frame 16711422 {
        }
        frame 1535 {
        }
        frame 2621184 {
        }
      }
      n565 = case shown="2621184" w770 {
        tunnel: [404 1 3 2 0 5 4] -> w703
        frame Default {
        }
        frame 16711686 {
        }
        frame 15728450 {
        }
        frame 16752640 {
        }
        frame 16711422 {
        }
        frame 1535 {
        }
        frame 2621184 {
        }
      }
      n566 = case shown="2621184" w782 {
        tunnel: [404 1 3 2 0 5 4] -> w729
        frame Default {
        }
        frame 16711686 {
        }
        frame 15728450 {
        }
        frame 16752640 {
        }
        frame 16711422 {
        }
        frame 1535 {
        }
        frame 2621184 {
        }
      }
      n567 = case shown="2621184" w785 {
        tunnel: [404 1 3 2 0 5 4] -> w726
        frame Default {
        }
        frame 16711686 {
        }
        frame 15728450 {
        }
        frame 16752640 {
        }
        frame 16711422 {
        }
        frame 1535 {
        }
        frame 2621184 {
        }
      }
      n568 = case shown="2621184" w774 {
        tunnel: [404 1 3 2 0 5 4] -> w719
        frame Default {
        }
        frame 16711686 {
        }
        frame 15728450 {
        }
        frame 16752640 {
        }
        frame 16711422 {
        }
        frame 1535 {
        }
        frame 2621184 {
        }
      }
      n569 = case shown="2621184" w773 {
        tunnel: [404 1 3 2 0 5 4] -> w716
        frame Default {
        }
        frame 16711686 {
        }
        frame 15728450 {
        }
        frame 16752640 {
        }
        frame 16711422 {
        }
        frame 1535 {
        }
        frame 2621184 {
        }
      }
      n570 = case shown="2621184" w771 {
        tunnel: [404 1 3 2 0 5 4] -> w710
        frame Default {
        }
        frame 16711686 {
        }
        frame 15728450 {
        }
        frame 16752640 {
        }
        frame 16711422 {
        }
        frame 1535 {
        }
        frame 2621184 {
        }
      }
      n571 = case shown="2621184" w772 {
        tunnel: [404 1 3 2 0 5 4] -> w711
        frame Default {
        }
        frame 16711686 {
        }
        frame 15728450 {
        }
        frame 16752640 {
        }
        frame 16711422 {
        }
        frame 1535 {
        }
        frame 2621184 {
        }
      }
      n572 = case shown="2621184" w769 {
        tunnel: [404 1 3 2 0 5 4] -> w702
        frame Default {
        }
        frame 16711686 {
        }
        frame 15728450 {
        }
        frame 16752640 {
        }
        frame 16711422 {
        }
        frame 1535 {
        }
        frame 2621184 {
        }
      }
      n573 = case shown="2621184" w766 {
        tunnel: [404 1 3 2 0 5 4] -> w722
        frame Default {
        }
        frame 16711686 {
        }
        frame 15728450 {
        }
        frame 16752640 {
        }
        frame 16711422 {
        }
        frame 1535 {
        }
        frame 2621184 {
        }
      }
      n574 = case shown="1535" w767 {
        tunnel: [404 1 3 2 0 5 4] -> w721
        frame Default {
        }
        frame 16711686 {
        }
        frame 15728450 {
        }
        frame 16752640 {
        }
        frame 16711422 {
        }
        frame 1535 {
        }
        frame 2621184 {
        }
      }
      n575 = case shown="2621184" w761 {
        tunnel: [404 1 3 2 0 5 4] -> w705
        frame Default {
        }
        frame 16711686 {
        }
        frame 15728450 {
        }
        frame 16752640 {
        }
        frame 16711422 {
        }
        frame 1535 {
        }
        frame 2621184 {
        }
      }
      n576 = case shown="2621184" w765 {
        tunnel: [404 1 3 2 0 5 4] -> w718
        frame Default {
        }
        frame 16711686 {
        }
        frame 15728450 {
        }
        frame 16752640 {
        }
        frame 16711422 {
        }
        frame 1535 {
        }
        frame 2621184 {
        }
      }
      n577 = case shown="2621184" w764 {
        tunnel: [404 1 3 2 0 5 4] -> w715
        frame Default {
        }
        frame 16711686 {
        }
        frame 15728450 {
        }
        frame 16752640 {
        }
        frame 16711422 {
        }
        frame 1535 {
        }
        frame 2621184 {
        }
      }
      n578 = case shown="2621184" w757 {
        tunnel: [404 1 3 2 0 5 4] -> w700
        frame Default {
        }
        frame 16711686 {
        }
        frame 15728450 {
        }
        frame 16752640 {
        }
        frame 16711422 {
        }
        frame 1535 {
        }
        frame 2621184 {
        }
      }
      n579 = case shown="1535" w758 {
        tunnel: [404 1 3 2 0 5 4] -> w701
        frame Default {
        }
        frame 16711686 {
        }
        frame 15728450 {
        }
        frame 16752640 {
        }
        frame 16711422 {
        }
        frame 1535 {
        }
        frame 2621184 {
        }
      }
      n580 = case shown="2621184" w752 {
        tunnel: [404 1 3 2 0 5 4] -> w695
        frame Default {
        }
        frame 16711686 {
        }
        frame 15728450 {
        }
        frame 16752640 {
        }
        frame 16711422 {
        }
        frame 1535 {
        }
        frame 2621184 {
        }
      }
      n581 = case shown="2621184" w762 {
        tunnel: [404 1 3 2 0 5 4] -> w709
        frame Default {
        }
        frame 16711686 {
        }
        frame 15728450 {
        }
        frame 16752640 {
        }
        frame 16711422 {
        }
        frame 1535 {
        }
        frame 2621184 {
        }
      }
      n582 = case shown="2621184" w763 {
        tunnel: [404 1 3 2 0 5 4] -> w712
        frame Default {
        }
        frame 16711686 {
        }
        frame 15728450 {
        }
        frame 16752640 {
        }
        frame 16711422 {
        }
        frame 1535 {
        }
        frame 2621184 {
        }
      }
      n583 = case shown="2621184" w760 {
        tunnel: [404 1 3 2 0 5 4] -> w704
        frame Default {
        }
        frame 16711686 {
        }
        frame 15728450 {
        }
        frame 16752640 {
        }
        frame 16711422 {
        }
        frame 1535 {
        }
        frame 2621184 {
        }
      }
      n584 = case shown="2621184" w756 {
        tunnel: [404 1 3 2 0 5 4] -> w699
        frame Default {
        }
        frame 16711686 {
        }
        frame 15728450 {
        }
        frame 16752640 {
        }
        frame 16711422 {
        }
        frame 1535 {
        }
        frame 2621184 {
        }
      }
      n585 = case shown="2621184" w755 {
        tunnel: [404 1 3 2 0 5 4] -> w698
        frame Default {
        }
        frame 16711686 {
        }
        frame 15728450 {
        }
        frame 16752640 {
        }
        frame 16711422 {
        }
        frame 1535 {
        }
        frame 2621184 {
        }
      }
      n586 = case shown="2621184" w753 {
        tunnel: [404 1 3 2 0 5 4] -> w696
        frame Default {
        }
        frame 16711686 {
        }
        frame 15728450 {
        }
        frame 16752640 {
        }
        frame 16711422 {
        }
        frame 1535 {
        }
        frame 2621184 {
        }
      }
      n587 = case shown="2621184" w754 {
        tunnel: [404 1 3 2 0 5 4] -> w697
        frame Default {
        }
        frame 16711686 {
        }
        frame 15728450 {
        }
        frame 16752640 {
        }
        frame 16711422 {
        }
        frame 1535 {
        }
        frame 2621184 {
        }
      }
      n588 = case shown="2621184" w751 {
        tunnel: [404 1 3 2 0 5 4] -> w694
        frame Default {
        }
        frame 16711686 {
        }
        frame 15728450 {
        }
        frame 16752640 {
        }
        frame 16711422 {
        }
        frame 1535 {
        }
        frame 2621184 {
        }
      }
      n589 = case shown="2621184" w748 {
        tunnel: [404 1 3 2 0 5 4] -> w723
        frame Default {
        }
        frame 16711686 {
        }
        frame 15728450 {
        }
        frame 16752640 {
        }
        frame 16711422 {
        }
        frame 1535 {
        }
        frame 2621184 {
        }
      }
      n590 = case shown="1535" w749 {
        tunnel: [404 1 3 2 0 5 4] -> w720
        frame Default {
        }
        frame 16711686 {
        }
        frame 15728450 {
        }
        frame 16752640 {
        }
        frame 16711422 {
        }
        frame 1535 {
        }
        frame 2621184 {
        }
      }
      n591 = case shown="2621184" w743 {
        tunnel: [404 1 3 2 0 5 4] -> w707
        frame Default {
        }
        frame 16711686 {
        }
        frame 15728450 {
        }
        frame 16752640 {
        }
        frame 16711422 {
        }
        frame 1535 {
        }
        frame 2621184 {
        }
      }
      n592 = case shown="2621184" w747 {
        tunnel: [404 1 3 2 0 5 4] -> w717
        frame Default {
        }
        frame 16711686 {
        }
        frame 15728450 {
        }
        frame 16752640 {
        }
        frame 16711422 {
        }
        frame 1535 {
        }
        frame 2621184 {
        }
      }
      n593 = case shown="2621184" w746 {
        tunnel: [404 1 3 2 0 5 4] -> w714
        frame Default {
        }
        frame 16711686 {
        }
        frame 15728450 {
        }
        frame 16752640 {
        }
        frame 16711422 {
        }
        frame 1535 {
        }
        frame 2621184 {
        }
      }
      n594 = case shown="2621184" w744 {
        tunnel: [404 1 3 2 0 5 4] -> w708
        frame Default {
        }
        frame 16711686 {
        }
        frame 15728450 {
        }
        frame 16752640 {
        }
        frame 16711422 {
        }
        frame 1535 {
        }
        frame 2621184 {
        }
      }
      n595 = case shown="2621184" w745 {
        tunnel: [404 1 3 2 0 5 4] -> w713
        frame Default {
        }
        frame 16711686 {
        }
        frame 15728450 {
        }
        frame 16752640 {
        }
        frame 16711422 {
        }
        frame 1535 {
        }
        frame 2621184 {
        }
      }
      n596 = case shown="2621184" w742 {
        tunnel: [404 1 3 2 0 5 4] -> w706
        frame Default {
        }
        frame 16711686 {
        }
        frame 15728450 {
        }
        frame 16752640 {
        }
        frame 16711422 {
        }
        frame 1535 {
        }
        frame 2621184 {
        }
      }
      n597 = Build Array(w741, w739, w740, w738, 0 ("element"), w737, w736, w734, w735) -> (w691:i32[])
      n598 = Build Array(w732, w730, w731, w733, 1 ("element"), w729, w728, w726, w727) -> (w692:i32[])
      n599 = Build Array(w724, w716, w719, w725, 5 ("element"), w711, w710, w702, w703) -> (w693:i32[])
      n600 = Build Array(w722, w715, w718, w721, 3 ("element"), w712, w709, w704, w705) -> (w690:i32[])
      n601 = Build Array(w695, w694, w696, w697, 2 ("element"), w701, w699, w698, w700) -> (w689:i32[])
      n602 = Build Array(w723, w714, w717, w720, 4 ("element"), w713, w708, w706, w707) -> (w688:i32[])
      n603 = Build Array(w692, w693, w689, w688, w691, w690) -> (w796:i32[][])
    }
  }
  "Array" <- w1
